vi "Dashboard Main0.vi"() -> ()   [LabVIEW 2015]
uses:
  Vision FRC Color Processing Example Folder - Copy/Vision Support Code/Camera Types.ctl
  <vilib>/Utility/miscctls.llb/LVRowAndColumnTypeDef.ctl
  <vilib>/event_ctls.llb/eventvkey.ctl
  <vilib>/Rock Robotics/Network Tables/NT Read Boolean.vi
  <vilib>/Rock Robotics/Network Tables/NT Write Boolean.vi
  <vilib>/Rock Robotics/WPI/Dashboard/WPI_DashboardLogging Global.vi
  <vilib>/Utility/config.llb/Write Key (String).vi
  <vilib>/Utility/config.llb/Write Key (I32).vi
  <vilib>/Rock Robotics/Network Tables/NT Read Numeric Array.vi
  <vilib>/Utility/config.llb/NI_LVConfig.lvlib
panel:
  out "Auton Finished 2":bool=TRUE
  in  "Camera Type":T1=enum."MS HD3000 square"
  in  "TCP":refnum<k5>
  in  "Rec Mode":enum32{"Stop", "Record", "Playback"}(radio)
  in  "Vision":u16(ring) items=["Camera Off", "USB Camera SW", "USB Camera HW", "IP Camera"]
  out "Camera IP":string
  out "Image Message":string="Timeout in Camera Communications"
  in  "Dashboard Tab":T2(tab)=enum."Custom"
  out "Shoot Now":bool=TRUE
  in  "Shoot":bool
  in  "Defense Type":T3(ring)
  out "Auton Finished":bool
  in  "Camera Switch":bool
  out "NT Connection":bool
  in  "Camera Settings":T4={"Frame Rate"=30, "Compression"=30, "Size"=1} {"Frame Rate" scale=1.0..30.0; "Size" items=["640x480", "320x240", "160x120"]}
  out "Mode":T5(ring)=enum."Auto Disabled"
  in  "DB Camera Config":bool
  out "fps":dbl format="%#.1g"
  out "Mbps":dbl format="%#.1g"
  out "Mbps LED":bool
  out "RPM":dbl(slide) scale=0.0..20000.0
  out "Arm Encoder":dbl(slide) scale=-1.0..1.0
  out "Camera Aimed":bool
  in  "Defense Location":enum16{"0", "1", "2", "3", "4", "5"}(ring)
  out "Shooter Current":dbl(graph)
  in  "DB/String 0":string
  in  "DB/Slider 1":dbl(slide) scale=0.0..5.0
  out "DB/LED 1":bool
  out "DB/LED 0":bool
  in  "DB/Button 3":bool
  in  "DB/Button 2":bool
  in  "DB/Button 1":bool caption="LED Light"
  in  "DB/Button 0":bool
  out "JS1 Z":dbl(slide) scale=-1.0..1.0 scale format="%#_2e"
  out "JS1 Graph":cluster{"X":dbl, "Y":dbl}[](graph)
  out "JS1 Buttons":T6
  out "JS2 Z":dbl(slide) scale=-1.0..1.0 scale format="%#_2e"
  out "JS2 Graph":cluster{"X":dbl, "Y":dbl}[](graph)
  out "JS2 Buttons":T6
  out "Detected Targets":T7(array[cluster]) {"Normalized Rect"."Numeric 5" format="%#_2g"; "Normalized Rect"."Numeric 3" format="%#_2g"; "Normalized Rect"."Numeric 2" format="%#_2g"; "Normalized Rect"."Numeric" format="%#_2g"}
  in  "LED Color":T8={"Hue"={51.43401092766074, 170.53085495574481}, "Sat"={34.78571428571429, 255.0}, "Val"={91.07142857142858, 255.0}} {"Hue" scale=0.0..255.0 scale format="%#_3g"}
  in  "Std Devs for Calibration":cluster{"H":dbl, "S":dbl, "V":dbl}={"H"=4.0, "S"=6.0, "V"=6.0}
  in  "Min Score Threshold":i32=20
  out "Target Distance":dbl
  out "Target X":dbl
  out "Target Y":dbl
  in  "Test Slider":dbl(slide) scale=0.0..100.0 scale format="%#_3g"
  in  "On/Off":bool caption="Solenoid"
  in  "Test Name":u16(ring) items=["Select the test to run..."]
  in  "Test Tree":string(tree)
  in  "Motor":cluster{"Value":dbl, "Enable":bool} {"Value" scale=-1.0..1.0 scale format="%#_3g"}
  out "Progress":T9 {"Test Progress" scale=0.0..100.0}
  in  "Rev/Fwd":cluster{"Forward":bool, "Reverse":bool}
  in  "Test Ring":u16(ring) items=["Monochrome", "Color"]
  out "Cmd Status":string
  in  "Execute Command":bool
  in  "Command Params":string[][](table)
  in  "Command Selection":i32(listbox)
  in  "CheckList":i32(listbox)
  out "Tree":string(tree)
  out "Camera Image":T10(plugin-control)
  out "Background":bool
  # "Right"
  # "Left"
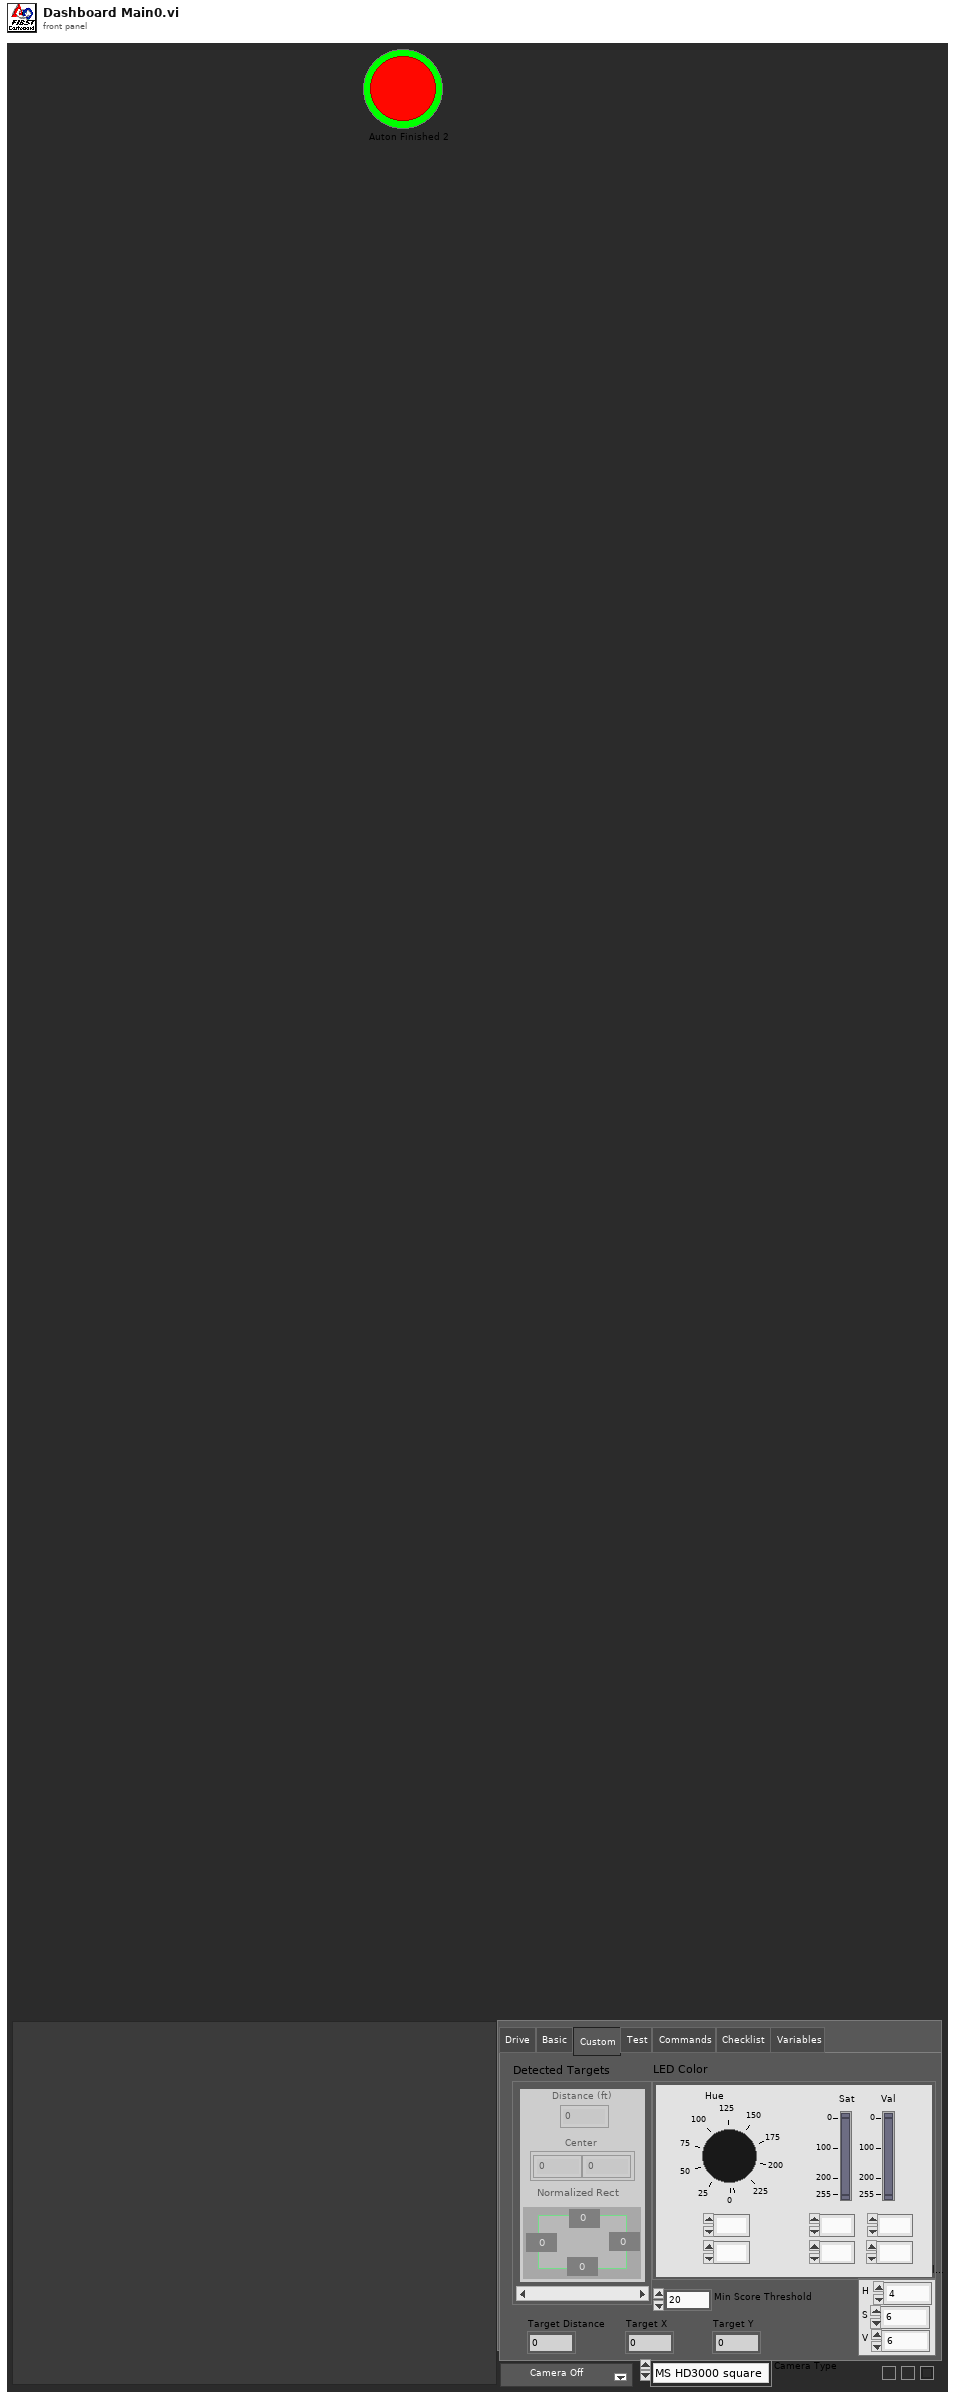
[diagram p1: front panel]
types:
  T1 = typedef "Camera Types.ctl" = enum16{"206", "1011", "1013", "MS HD3000 square", "MS HD3000 640x480"}
  T2 = enum32{"Drive", "Basic", "Custom", "Test", "Commands", "Checklist", "Variables"}
  T3 = enum16{"None", "Rampart", "Moat", "Rock Wall", "Rough Terrain", "Low Bar", "Chili Fries"}
  T4 = cluster{"Frame Rate":i32, "Compression":i32, "Size":u16}
  T5 = enum8{"Tele-Op Disabled", "Tele-Op Enabled", "Auto Disabled", "Auto Enabled", "Test Disabled", "Test Enabled", "Disconnected", "No Code", "E-Stop"}
  T6 = cluster{bool, bool, bool, bool, bool, bool, bool, bool, bool, bool, bool, bool}
  T7 = cluster{"Distance (ft)":dbl, "Center":cluster{dbl, dbl}, "Normalized Rect":cluster{"Numeric":dbl, "Numeric 2":dbl, "Numeric 3":dbl, "Numeric 5":dbl}}[]
  T8 = cluster{"Hue":cluster{dbl, dbl}, "Sat":cluster{dbl, dbl}, "Val":cluster{dbl, dbl}}
  T9 = cluster{"Test Progress":u8, "Test Progress Text":string}
  T10 = typedef "IMAQ Image.ctl" = refnum<image>
  T11 = cluster{"IDs":cluster{"RPC field ID":u16, "Unique ID":u16}, "String":string}
  T12 = enum32{"Drive", "Basic", "Custom", "Test", "Checklist", "Variables"}
  T13 = typedef "Image Type" = u32
  T14 = cluster{"Camera Image":refnum<vi>, "Dashboard Tab":refnum<vi>, "Background":refnum<vi>, "Vision":refnum<vi>, "Rec Mode":refnum<vi>, "Test Slider":refnum<vi>, "On/Off ":refnum<vi>, "Test Ring":refnum<vi>, "Rev/Fwd":refnum<vi>, "Test Name":refnum<vi>, "Motor":refnum<vi>, "Progress":refnum<vi>, "CheckList":refnum<vi>, "Tree":refnum<vi>, "Test Tree":refnum<vi>, "Command Params":refnum<vi>, "Command Selection":refnum<vi>, "Execute Command":refnum<vi>, "Cmd Status":refnum<vi>}
  T15 = typedef "NI_LVConfig.lvlib/Config Data RefNum.ctl" = refnum<k1>
  T16 = enum16{"open", "open or create", "create or replace", "create", "open (read only)"}
  T17 = cluster{"Error Strings":string, "Disable Counts":cluster{u16, u16}, "Rail Faults":cluster{u16, u16, u16}, "Robot IP":string, "DB Mode":u8, "Event Info":cluster{"Name":string, "Type":u8, "Number":u16, "Replay":u8}, "Camera Addr":string}
  T18 = cluster{"Storage":cluster{"Disk Free":u64, "RAM Block":u32, "RAM free":u32}, "CPU Utilization":cluster{"CPU % ISR":sgl, "CPU % Time Crit":sgl, "CPU % Timed Str":sgl, "CPU % High":sgl, "CPU % Above":sgl, "CPU % Normal":sgl, "CPU % Low":sgl}, "CAN":cluster{"% Bus Utilization":sgl, "Bus Off Cnt":u32, "TX_FIFO Full Cnt":u32, "Receive Error Cnt":u8, "Transmit Error Cnt":u8}, "HID":cluster{"HID Outputs":u32, "Rumble Low":u16, "Rumble High":u16}[]}
  T19 = cluster{"Status bits":cluster{"Test Mode":bool, "Autonomous":bool, "Enabled":bool, "Code Start":bool, "Brownout":bool, "Reserved 2":bool, "Reserved 3":bool, "E-Stop":bool}, "Code Trace":cluster{"Disabled":bool, "TeleOp":bool, "Auto":bool, "Test":bool}, "Controller Type":enum16{"unknown", "cRIO", "roboRio"}, "Code?":enum16{"unknown", "noCode", "code"}, "Battery V":dbl}
  T20 = cluster{"Control Bits":cluster{"TestMode":bool, "Autonomous":bool, "Enabled":bool, "FMS Present":bool, bool, bool, bool, "E-Stop":bool}, "Team Station ":u8, "Countdown":sgl, "Joystick Values":cluster{"Axes":dbl[], "Buttons":bool[], "POVs":i16[]}[]}
  T21 = cluster{"Axes":dbl[], "Buttons":bool[], "POVs":i16[]}[]
  T22 = cluster{"Test Mode":bool, "Autonomous":bool, "Enabled":bool, "Code Start":bool, "Brownout":bool, "Reserved 2":bool, "Reserved 3":bool, "E-Stop":bool}
  T23 = cluster{"Axes":dbl[], "Buttons":bool[], "POVs":i16[]}
  T24 = cluster{"Buttons[0]":bool, "Buttons[1]":bool, "Buttons[2]":bool, "Buttons[3]":bool, "Buttons[4]":bool, "Buttons[5]":bool, "Buttons[6]":bool, "Buttons[7]":bool, "Buttons[8]":bool, "Buttons[9]":bool, "Buttons[10]":bool, "Buttons[11]":bool}
  T25 = cluster{"Detected Targets[0]":cluster{"Distance (ft)":dbl, "Center":cluster{dbl, dbl}, "Normalized Rect":cluster{"Numeric":dbl, "Numeric 2":dbl, "Numeric 3":dbl, "Numeric 5":dbl}}, "Detected Targets[1]":cluster{"Distance (ft)":dbl, "Center":cluster{dbl, dbl}, "Normalized Rect":cluster{"Numeric":dbl, "Numeric 2":dbl, "Numeric 3":dbl, "Numeric 5":dbl}}, "Detected Targets[2]":cluster{"Distance (ft)":dbl, "Center":cluster{dbl, dbl}, "Normalized Rect":cluster{"Numeric":dbl, "Numeric 2":dbl, "Numeric 3":dbl, "Numeric 5":dbl}}, "Detected Targets[3]":cluster{"Distance (ft)":dbl, "Center":cluster{dbl, dbl}, "Normalized Rect":cluster{"Numeric":dbl, "Numeric 2":dbl, "Numeric 3":dbl, "Numeric 5":dbl}}, "Detected Targets[4]":cluster{"Distance (ft)":dbl, "Center":cluster{dbl, dbl}, "Normalized Rect":cluster{"Numeric":dbl, "Numeric 2":dbl, "Numeric 3":dbl, "Numeric 5":dbl}}, "Detected Targets[5]":cluster{"Distance (ft)":dbl, "Center":cluster{dbl, dbl}, "Normalized Rect":cluster{"Numeric":dbl, "Numeric 2":dbl, "Numeric 3":dbl, "Numeric 5":dbl}}, "Detected Targets[6]":cluster{"Distance (ft)":dbl, "Center":cluster{dbl, dbl}, "Normalized Rect":cluster{"Numeric":dbl, "Numeric 2":dbl, "Numeric 3":dbl, "Numeric 5":dbl}}, "Detected Targets[7]":cluster{"Distance (ft)":dbl, "Center":cluster{dbl, dbl}, "Normalized Rect":cluster{"Numeric":dbl, "Numeric 2":dbl, "Numeric 3":dbl, "Numeric 5":dbl}}, "Detected Targets[8]":cluster{"Distance (ft)":dbl, "Center":cluster{dbl, dbl}, "Normalized Rect":cluster{"Numeric":dbl, "Numeric 2":dbl, "Numeric 3":dbl, "Numeric 5":dbl}}}
  T26 = cluster{"Distance (ft)":dbl, "Center":cluster{dbl, dbl}, "Normalized Rect":cluster{"Numeric":dbl, "Numeric 2":dbl, "Numeric 3":dbl, "Numeric 5":dbl}}
  T27 = cluster{"Numeric":dbl, "Numeric 2":dbl, "Numeric 3":dbl, "Numeric 5":dbl}
  T28 = cluster{"Operation":enum16{"Update", "Clear"}, "Color Box":u32}[]
  T29 = typedef "eventvkey.ctl" = enum16{"ASCII", "Enter", "Return", "Shift", "Ctrl", "Alt", "Cmd", "Opt", "Caps", "NumLock", "Clear", "Break", "Up", "Down", "Left", "Right", "Insert", "Delete", "Home", "End", "PageUp", "PageDown", "Escape", "Help", "Pause", "ScrollLock", "F1", "F2", "F3", "F4", "F5", "F6", "F7", "F8", "F9", "F10", "F11", "F12", "F13", "F14", "F15", "F16", "F17", "F18", "F19", "F20", "F21", "F22", "F23", "F24", "Play", "VolumeUp", "VolumeDown", "Mute", "Two Byte Char"}
  T30 = cluster{"Image Size":bool, "Image Type":bool, "Pixel Value":bool, "ROI Information":bool, "Zoom Factor":bool}
  T31 = enum8{"Enabled", "Disabled", "Disabled and Grayed Out"}
  T32 = cluster{"Operation":enum16{"Update", "Clear"}, "Color Box":u32}
  T33 = typedef "LVRowAndColumnTypeDef.ctl" = cluster{"Row":i32, "Column":i32}
  T34 = cluster{"Shift":bool, "Ctrl":bool, "Alt":bool, "Cmd":bool, "Opt":bool}
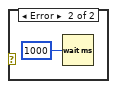
[diagram p2: hidden frame]
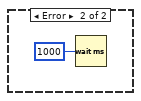
[diagram p3: hidden frame]
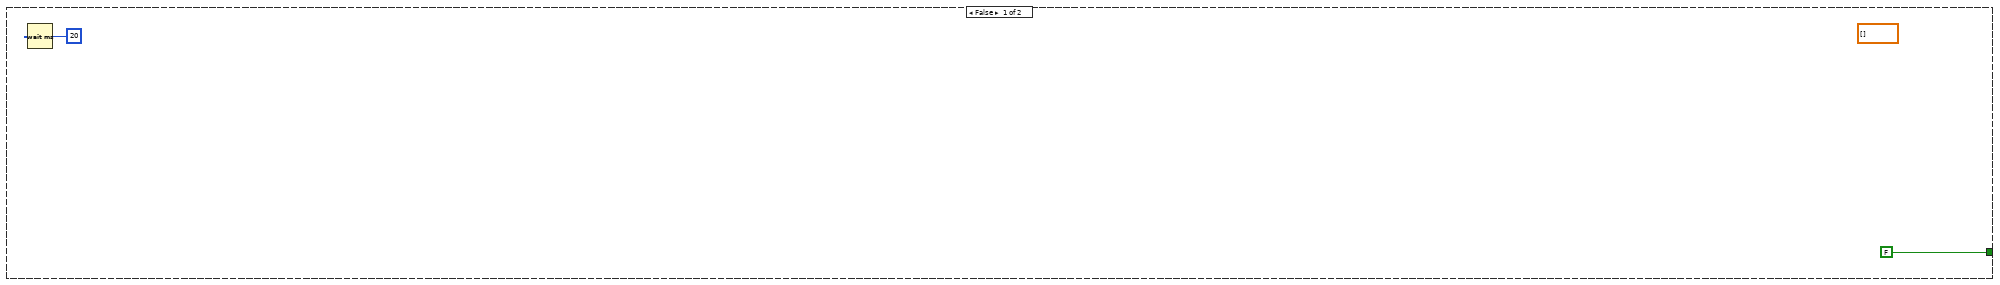
[diagram p4: hidden frame]
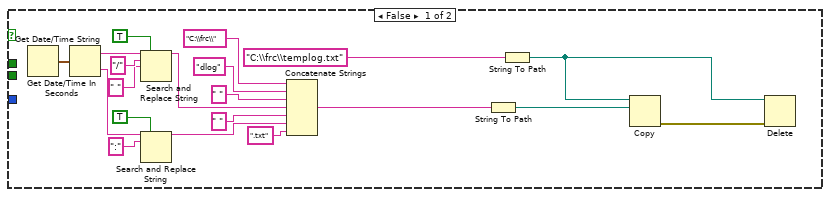
[diagram p5: hidden frame]
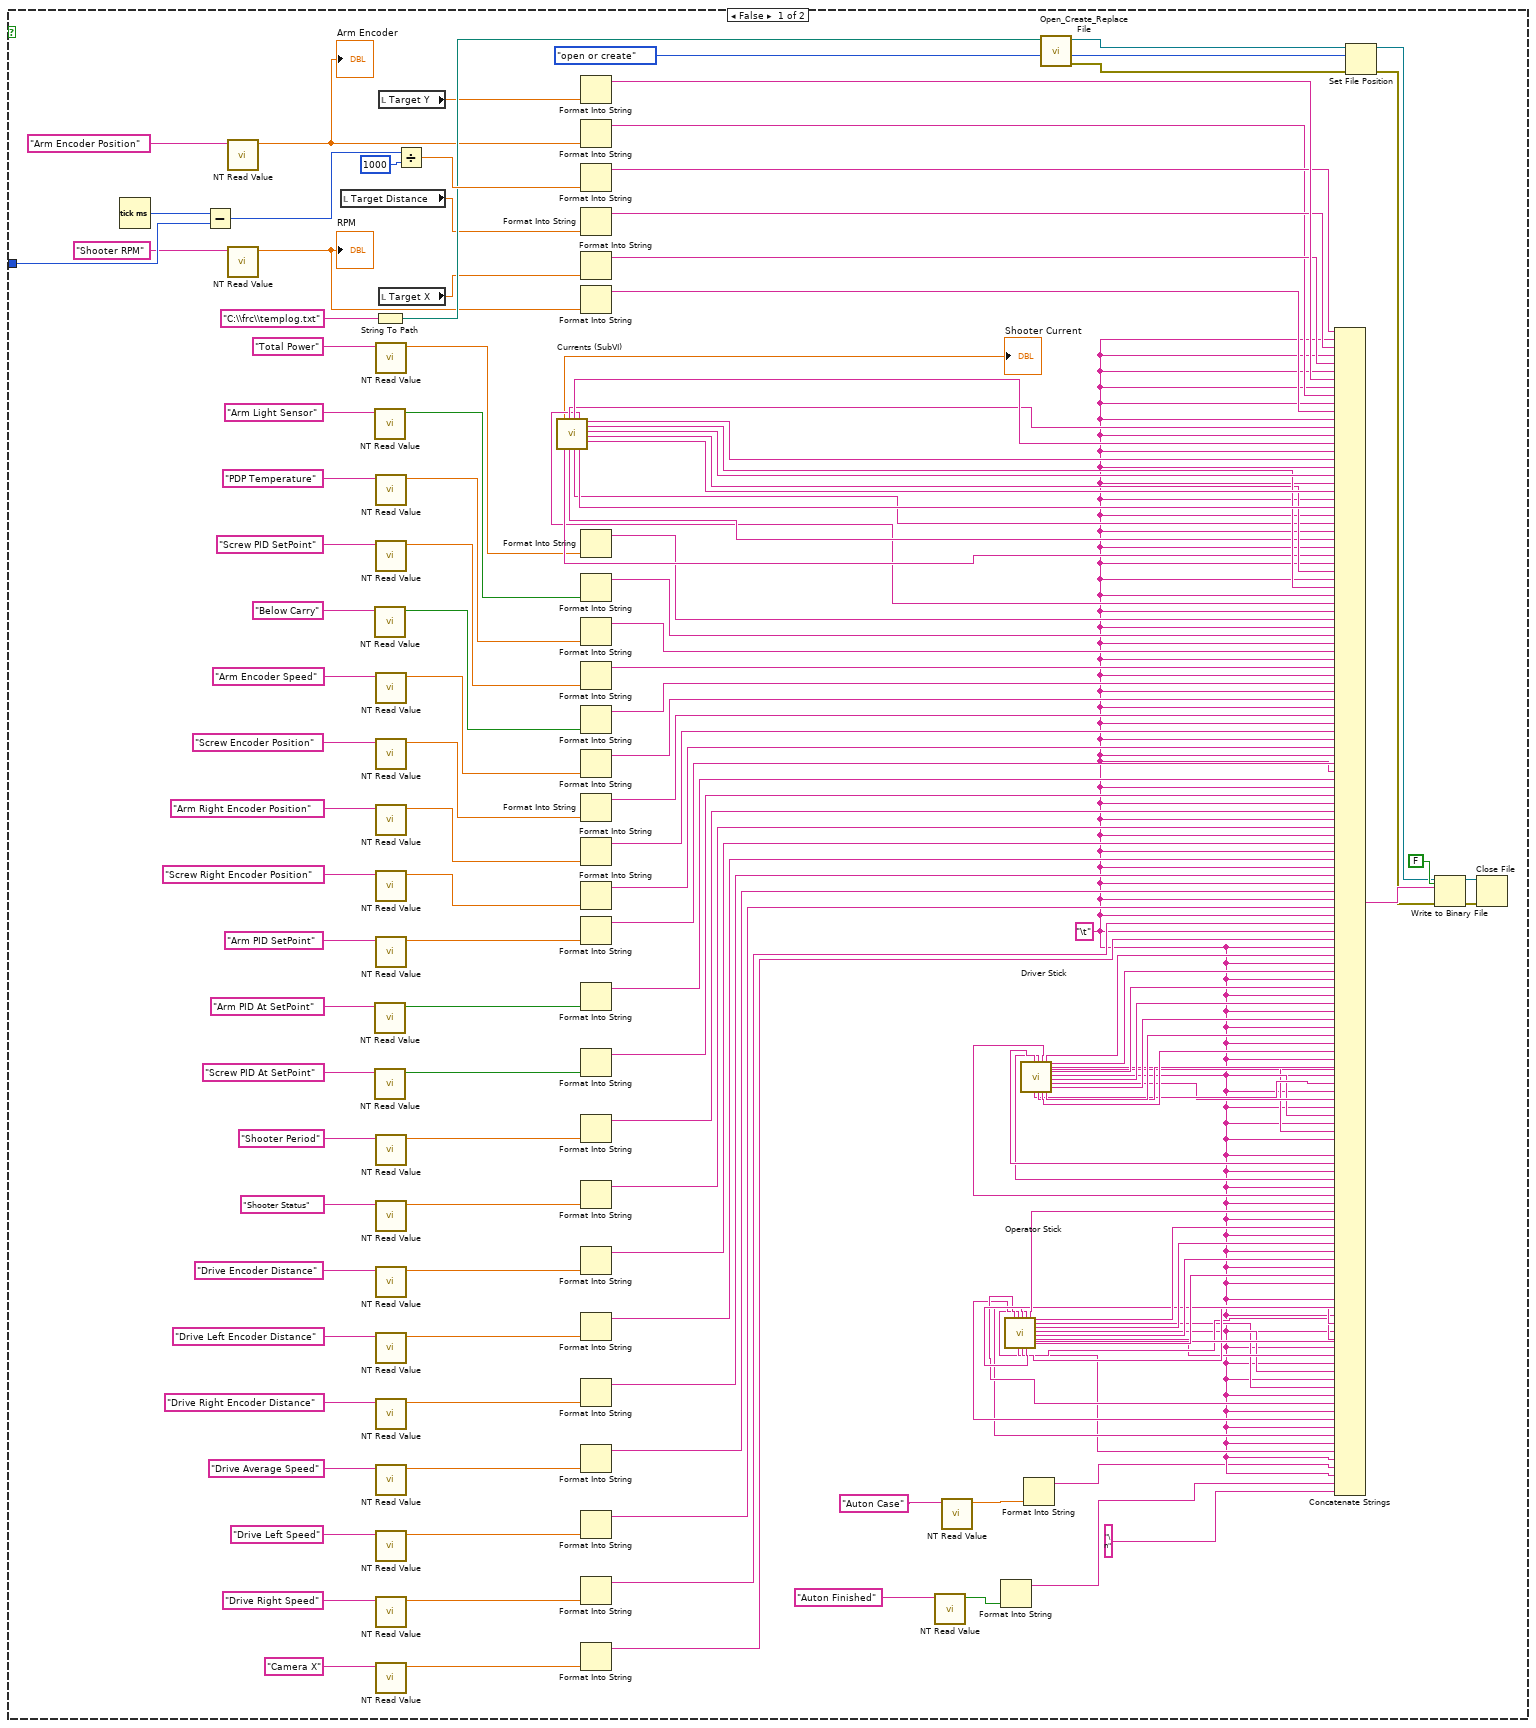
[diagram p6: hidden frame]
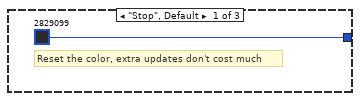
[diagram p7: hidden frame]
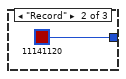
[diagram p8: hidden frame]
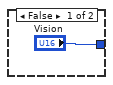
[diagram p10: hidden frame]
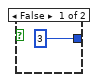
[diagram p11: hidden frame]
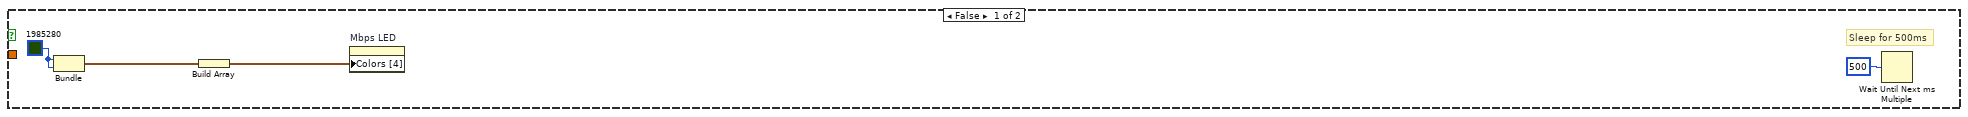
[diagram p12: hidden frame]
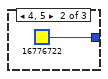
[diagram p13: hidden frame]
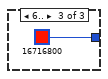
[diagram p14: hidden frame]
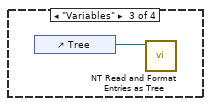
[diagram p16: hidden frame]
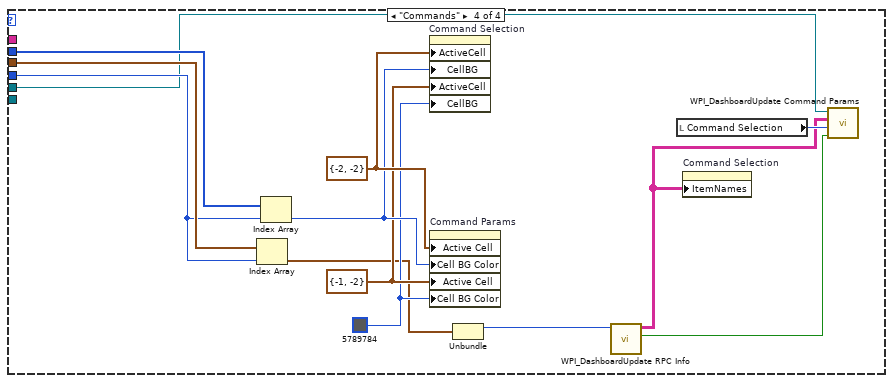
[diagram p17: hidden frame]
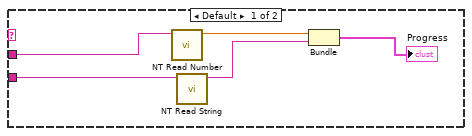
[diagram p18: hidden frame]
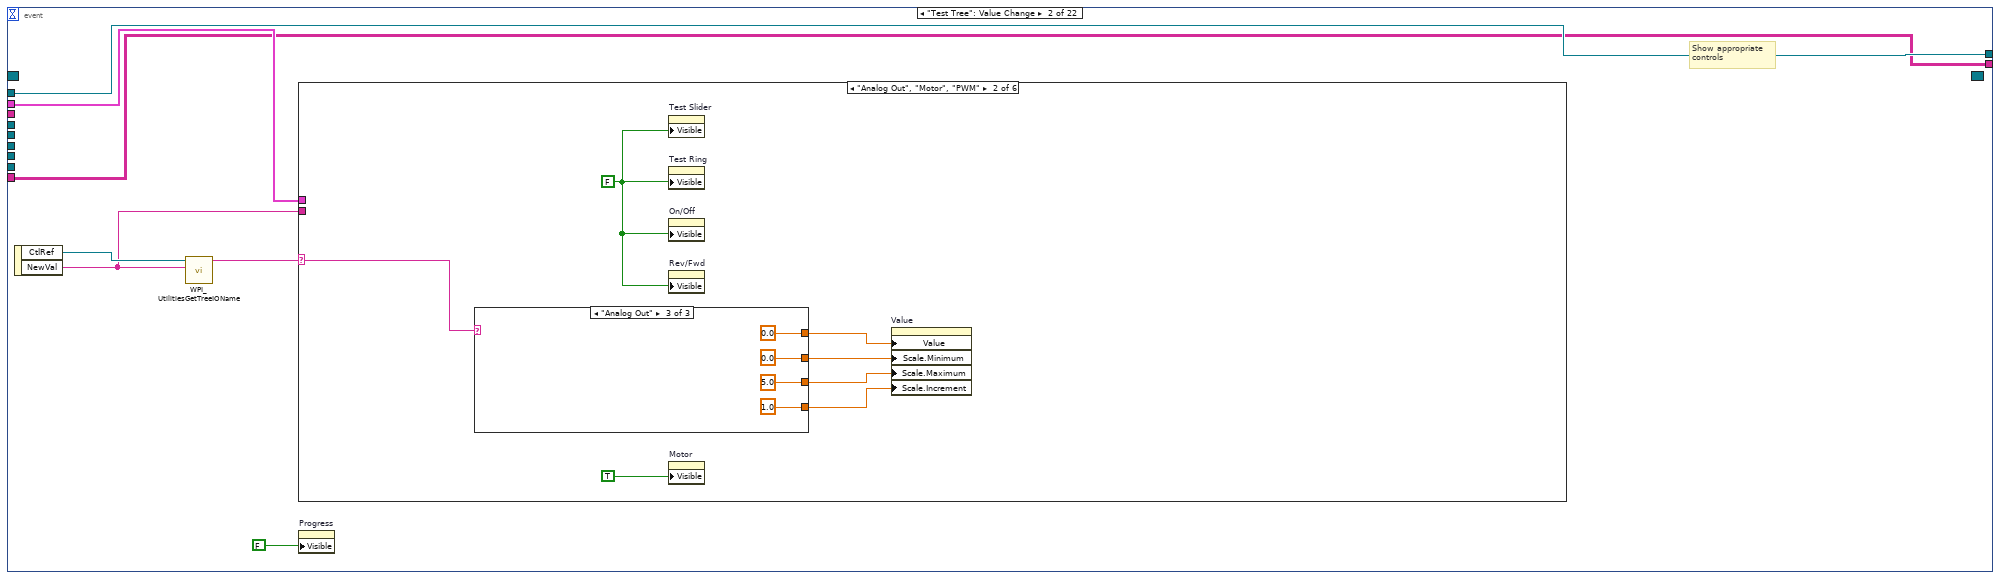
[diagram p19: hidden frame]
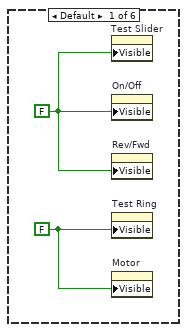
[diagram p20: hidden frame]
diagram:
  w10 = T11 {"IDs"={"RPC field ID"=0, "Unique ID"=0}, "String"=""}  # RPC Response
  w34 = 491  # min tab size
  w33 = 1.333  # min tab size
  w42 = enum32{"Stop", "Record", "Playback"}."Stop" ("Rec Mode")
  w16 = FALSE ("Visible")
  (unwired) "This VI has seven parallel loops for different tasks and a bit of initialization code that runs just once.\n\nTypical dashboard extensions only need to edit the panel. Adding new indicators or controls simply involves placing them on the panel in the Operations tab and naming them the same as the SmartDashboard variable on the robot\n\nIf the display needs to process the data before display, loop one is an example of doing that for the joysticks and motors.\n\nIf you want customize the video display or perform processing on it, loop two is where that takes place.\n\nOther loops should not need to be modified. They are pretty standard, and document the task they perform."  # Documentation
  w62 = T13 4 items=["Grayscale (U8)", "Grayscale (I16)", "Grayscale (SGL)", "Complex (CSG)", "RGB (U32)", "HSL (U32)", "RGB (U64)"] ("Image Type")
  # "Loop 7. Wait for DS connections"
  # "Basic debug and auto controls: Their data names are fixed, but\nthe displayed name, called a caption, can be changed directly or in\nrobot code such as shown in Begin."
  # "Controls for Test Mode, Camera Settings, etc."
  # "Additional UI Initialization"
  # "Loop 6. Animation for background of window during playback and record"
  # "Fires each time robot IP\nchanges, simulator does this"
  # "Fires each time window\ndocking changes."
  # "Collects all controls and indicators\nin the Basic and Custom tab.\nIf you need to bind additional controls,\nadd their references. You can extend the\nenum constant or use an integer."
  # "The remaining code below this line typically doesn't need to be modified."
  # "Loop 4. Process UI events related to test mode, checklist, and camera settings"
  # "Terminals of controls and indicators that are bound to the smart dashboard by name.\nYou can place the terminals anywhere you like and even read data from them.\nYou bind controls by adding the control reference to the array on the left. The subVI will\ndo this for the contents of a tab, and you can do it for individual items too, as shown with\nthe LED. To create get the reference, right-click and Create>>Reference."
  # "Loop 3. Wait until the robot response provides\n the Robot IP address.\nOnce known, bind controls and\nvariables with the same names."
  # "Loop 5. Adjusts placement onscreen, hides the titlebar, etc."
  # "Loop 1. Receive various data streams from Driver Station, update joystick, motors, and more complex displays that don't easily bind to variables."
  # "Loop 2. Receive camera images from Robot, update Mbps, fps, and do any processing or display"
  n1 = control-ref of="Dashboard Tab"() -> (w40:refnum<vi>)
  n2 = control-ref of="Rec Mode"() -> (w22:refnum<vi>)
  n3 = control-ref of="Command Selection"() -> (w9:refnum<vi>)
  n4 = control-ref of="Command Params"() -> (w12:refnum<vi>)
  n5 = control-ref of="Execute Command"() -> (w11:refnum<vi>)
  n6 = control-ref of="Camera Image"() -> (w37:refnum<vi>)
  n7 = call "IMAQ Create"("Image Name"="Dashboard Image", "Image Type"=w62) -> ("New Image"=w60:T10, "error out"=w59:errorcluster)  [unwired: 2 in, 1 out]
  n8 = control-ref of="Dashboard Tab"() -> (w36:refnum<vi>)
  n9 = control-ref of="Tree"() -> (w26:refnum<vi>)
  n10 = control-ref of="Test Tree"() -> (w25:refnum<vi>)
  n11 = control-ref of="Background"() -> (w31:refnum<vi>)
  n12 = control-ref of="Cmd Status"() -> (w5:refnum<vi>)
  n13 = control-ref of="On/Off"() -> (w20:refnum<vi>)
  n14 = control-ref of="Test Name"() -> (w24:refnum<vi>)
  n15 = control-ref of="Command Params"() -> (w4:refnum<vi>)
  n16 = control-ref of="Test Slider"() -> (w21:refnum<vi>)
  n17 = control-ref of="Rev/Fwd"() -> (w18:refnum<vi>)
  n18 = control-ref of="Motor"() -> (w23:refnum<vi>)
  n19 = control-ref of="Progress"() -> (w17:refnum<vi>)
  n20 = control-ref of="CheckList"() -> (w27:refnum<vi>)
  n21 = control-ref of="Test Ring"() -> (w19:refnum<vi>)
  n22 = Obtain Notifier(name (unnamed)="Window Mode", notification data type=TRUE) -> (notifier out=w3:refnum<notifier>)  [unwired: 2 in, 2 out]
  n23 = call <vilib>:"Get Tab Control Refs.vi"("Page Index"=T12."Basic" ("Dashboard Tab"), "TabControl in"=w40) -> ("ControlsOnPage"=w15:refnum<vi>[])  [unwired: 9 in]
  n24 = call <vilib>:"Get Tab Control Refs.vi"("Page Index"=T12."Custom" ("Dashboard Tab"), "TabControl in"=w40) -> ("ControlsOnPage"=w39:refnum<vi>[])  [unwired: 9 in]
  n25 = control-ref of="Vision"() -> (w35:refnum<vi>)
  n26 = Bundle("min tab size"=w34, "min tab size"=w33) -> (w32:cluster{"min tab size":i32, "min tab size":dbl})  [unwired: 1 in]
  n27 = Obtain Notifier(name (unnamed)="Robot IP Update", notification data type="IP Addr" ("name (unnamed)")) -> (notifier out=w2:refnum<notifier>)  [unwired: 2 in, 2 out]
  n28 = property class="VI" props=["Front Panel.Closeable"]() -> (reference out=w41:refnum<vi>)  [unwired: 2 in, 2 out]
  n29 = vi-ref "Playback Controls.vi"() -> (w47:refnum<vi>)
  n30 = Build Array (concatenate)(w15, w39) -> (w38:refnum<vi>[])
  n31 = Bundle("Camera Image"=w37, "Dashboard Tab"=w36, "Background"=w31, "Vision"=w35, "Rec Mode"=w22, "Test Slider"=w21, "On/Off"=w20, "Test Ring"=w19, "Rev/Fwd"=w18, "Test Name"=w24, "Motor"=w23, "Progress"=w17, "CheckList"=w27, "Tree"=w26, "Test Tree"=w25, "Command Params"=w12, "Command Selection"=w9, "Execute Command"=w11, "Cmd Status"=w5) -> (w28:T14)  [unwired: 1 in]
  n32 = Create User Event(user event datatype=w10) -> (user event=w6:refnum<user-event>)  [unwired: 1 in, 1 out]
  n33 = call "Adjust Dashboard Window.vi"("Sizing Refnums"=w28, "Size Constraints"=w32, "VI"=w41, "WIn Mode"=w3) -> ()  [unwired: 8 in]
  n34 = while {
    tunnel: w38 -> [w75]
    tunnel: w2 -> [w73]
    tunnel: [w71] -> _
    tunnel: u32 1000 ("milliseconds to wait") -> [w70]
    tunnel: w6 -> [w63]
    i -> [w71]
    stop <- FALSE stop-if-true
    n35 = local read "Rec Mode"() -> (w66:enum32{"Stop", "Record", "Playback"})
    n36 = Wait on Notification(notifier=w73, timeout in ms (-1)=w70) -> (notification=w72:string, timed out?=w68:bool)  [unwired: 2 in, 2 out]
    n37 = Equal?(x=w66, y=u16 2 ("Rec Mode")) -> (x = y?=w67:bool)
    n38 = Compound Arithmetic op=OR(invert w68, w67) -> (w69:bool)
    n39 = case shown="True" w69 {
      tunnel: w75 -> [_ w79]
      tunnel: w72 -> [_ w78]
      tunnel: "Dashboard" -> [_ w77]
      tunnel: w63 -> [_ w76]
      frame False {
      }
      frame True {
        n40 = call <vilib>:"Bind Controls to SmartDashboard.vi"("RPC ref"=w76, "Client Name"=w77, "Bound Control Refs"=w79, "Server IP Address"=w78) -> ()  [unwired: 8 in]
      }
    }
  }
  n41 = register-events(refnum<vi> refnum, w6) -> (reference out=w46:refnum<event-registration>, error out=w45:errorcluster)  [unwired: 2 in]
  n42 = property class="VI"() -> ("Panel"=w49:refnum<vi>)  [unwired: 2 in, 2 out]
  n43 = call "Initialize Camera and CheckList.vi"("ListBox in"=w27) -> ("Cluster"=w53:cluster{"value":i32, "value":i32, "index":i32}, "Array"=w54:cluster{string[]}[], "File Refnum"=w52:T15)  [unwired: 8 in]
  n44 = property class="Pnl"(reference=w49) -> ("Panes[]"=w50:refnum<vi>[])  [unwired: 1 in, 2 out]
  n45 = property on="Camera Settings" class="Clust (strict)"("Val(Sgnl)"=w53) -> ()  [unwired: 2 in, 2 out]
  n46 = Tick Count (ms)() -> (millisecond timer value=w1:u32)
  n47 = control-ref of="Test Tree"() -> (w51:refnum<vi>)
  n48 = Index Array(array=w50) -> (element=w48:refnum<vi>)  [unwired: 1 in]
  n49 = while {
    tunnel: w48 -> [w81]
    i -> [w84]
    stop <- FALSE stop-if-true
    n50 = Wait (ms)(milliseconds to wait=u32 100) -> ()  [unwired: 1 out]
    n51 = case shown="\"Playback\"" "Rec Mode" {
      tunnel: w84 -> [_ _ w99]
      tunnel: [u32 2829099 ("Base Color") u32 11141120 ("Target Color") w88] -> w80
      frame "Stop", Default {
        # "Reset the color, extra updates don't cost much"
      }
      frame "Record" {
      }
      frame "Playback" {
        # "Playback"
        n52 = Quotient & Remainder(x=w99, y=u32 50 ("milliseconds to wait")) -> (x-y*floor(x/y)=w95:u32)  [unwired: 1 out]
        n53 = Divide(x=w95, y=u32 50 ("milliseconds to wait")) -> (x/y=w92:dbl)
        n54 = Multiply(x=6.283185307179586, y=w92) -> (x*y=w97:dbl)
        n55 = Sine(x=w97) -> (sin(x)=w96:dbl)
        n56 = Absolute Value(x=w96) -> (abs(x)=w89:dbl)
        n57 = call "Interpolate RGB Color.vi"("Proportion"=w89, "Target Color"=u32 30976, "Base Color"=u32 2829099) -> ("Result Color"=w88:u32)  [unwired: 8 in]
      }
    }
    n58 = property class="Pane"(reference=w81, "PaneColor"=w80) -> ()  [unwired: 1 in, 2 out]
  }
  n59 = while {
    tunnel: [w114] -> _
    tunnel: w2 -> [w108]
    tunnel: w15 -> [w107]
    tunnel: w3 -> [w103]
    tunnel: w1 -> [w102]
    shift-right: [w101] -> _
    shift-left: _ -> [w100]
    i -> [w114]
    stop <- FALSE stop-if-true
    n60 = call <vilib>:"WPI_DashboardUpdateNames.vi"("Controls on Tab"=w107) -> ()  [unwired: 11 in]
    n61 = local read "Vision"() -> (w105:u16)
    n62 = call <vilib>:"WPI_DashboardRetrieveStatusInfo.vi"("Vision"=w105, "Binding Refnum"=w108, "Window Mode Notifier"=w103, "TCP Cnx"="TCP") -> ("Power and Errors"=w109:T17, "Robot Metrics"=w112:T18, "Status Info"=w113:T19, "Control Info"=w110:T20, "Robot Mode"=w106:T5, "Process?"=w111:bool)  [unwired: 2 in]
    "Mode" <- w106
    n63 = case shown="True" w111 {
      tunnel: w113 -> [_ w143]
      tunnel: w112 -> [_ w142]
      tunnel: w110 -> [_ w141]
      tunnel: w109 -> [_ w140]
      tunnel: w106 -> [_ _]
      tunnel: w102 -> [_ w124]
      tunnel: [FALSE ("Enabled") w122] -> w101
      tunnel: w100 -> [_ w123]
      frame False {
        (unwired) dbl[] []
        n64 = Wait (ms)(milliseconds to wait=u32 20) -> ()  [unwired: 1 out]
      }
      frame True {
        # "swap motors to match\ncharts and include battery"
        n65 = Unbundle By Name(w141) -> ("Joystick Values"=w137:T21)  [unwired: 5 out]
        n66 = Unbundle By Name(w142) -> ()  [unwired: 5 out]
        n67 = Unbundle By Name(w140) -> ("Camera Addr"=→"Camera IP":string)  [unwired: 4 out]
        n68 = Unbundle By Name(w143) -> ("Status bits"=w125:T22)  [unwired: 1 out]
        n69 = Unbundle By Name(w125) -> ("Enabled"=w122:bool)  [unwired: 7 out]
        n70 = Index Array(array=w137) -> (element #1=w136:T23, element #2=w131:T23)  [unwired: 2 in]
        n71 = case shown="True" w122 {
          tunnel: w124 -> [_ w167]
          tunnel: w123 -> [_ w165]
          tunnel: w122 -> [_ w164]
          frame False {
            n72 = Get Date/Time In Seconds() -> (seconds since 1Jan1904=w156:timestamp)
            n73 = Get Date/Time String(seconds (now)=w156) -> (date string=w154:string, time string=w155:string)  [unwired: 2 in]
            n74 = Search and Replace String(replace all?=TRUE ("replace all? (F)"), input string=w154, search string="/", replace string=" " ("replace string (\"\")")) -> (result string=w147:string)  [unwired: 4 in, 3 out]
            n75 = Search and Replace String(replace all?=TRUE ("replace all? (F)"), input string=w155, search string=":") -> (result string=w145:string)  [unwired: 5 in, 3 out]
            n76 = Concatenate Strings("C:\\frc\\" ("string"), "dlog" ("string"), " " ("string"), w147, " " ("string"), w145, ".txt" ("string")) -> (w159:string)
            n77 = String To Path(string=w159) -> (path=w160:path)
            n78 = String To Path(string="C:\\frc\\templog.txt") -> (path=w161:path)
            n79 = Copy(10:w160, 11:w161) -> (0:w162:errorcluster)  [unwired: 3 in, 2 out]
            n80 = Delete(path (use dialog)=w161, error in=w162) -> ()  [unwired: 3 in, 3 out]
          }
          frame True {
            n81 = Not Equal?(x=w164, y=w165) -> (x != y?=w166:bool)
            n82 = case shown="True" w166 {
              tunnel: w167 -> [w281 _]
              frame False {
                w170 = "\t" ("string")
                n83 = Tick Count (ms)() -> (millisecond timer value=w283:u32)
                n84 = Subtract(x=w283, y=w281) -> (x-y=w282:u32)
                n85 = call-poly <vilib>:"NT Read Value.vi"("Name"="Arm Encoder Position") -> ("Numeric"=w276:dbl)  [unwired: 9 in, 1 out]
                "Arm Encoder" <- w276
                n86 = call-poly <vilib>:"NT Read Value.vi"("Name"="Shooter RPM") -> ("Numeric"=w273:dbl)  [unwired: 9 in, 1 out]
                "RPM" <- w273
                n87 = local read "Target Distance"() -> (w280:dbl)
                n88 = String To Path(string="C:\\frc\\templog.txt") -> (path=w293:path)
                n89 = call-poly <vilib>:"NT Read Value.vi"("Name"="Arm Light Sensor") -> ("Boolean"=w197:bool)  [unwired: 9 in, 1 out]
                n90 = call-poly <vilib>:"NT Read Value.vi"("Name"="Below Carry") -> ("Boolean"=w254:bool)  [unwired: 9 in, 1 out]
                n91 = call-poly <vilib>:"NT Read Value.vi"("Name"="Arm PID At SetPoint") -> ("Boolean"=w244:bool)  [unwired: 9 in, 1 out]
                n92 = call-poly <vilib>:"NT Read Value.vi"("Name"="Screw PID At SetPoint") -> ("Boolean"=w240:bool)  [unwired: 9 in, 1 out]
                n93 = call-poly <vilib>:"NT Read Value.vi"("Name"="Total Power") -> ("Numeric"=w269:dbl)  [unwired: 9 in, 1 out]
                n94 = call-poly <vilib>:"NT Read Value.vi"("Name"="PDP Temperature") -> ("Numeric"=w267:dbl)  [unwired: 9 in, 1 out]
                n95 = call-poly <vilib>:"NT Read Value.vi"("Name"="Screw PID SetPoint") -> ("Numeric"=w271:dbl)  [unwired: 9 in, 1 out]
                n96 = call-poly <vilib>:"NT Read Value.vi"("Name"="Arm Encoder Speed") -> ("Numeric"=w256:dbl)  [unwired: 9 in, 1 out]
                n97 = call-poly <vilib>:"NT Read Value.vi"("Name"="Screw Encoder Position") -> ("Numeric"=w260:dbl)  [unwired: 9 in, 1 out]
                n98 = call-poly <vilib>:"NT Read Value.vi"("Name"="Arm Right Encoder Position") -> ("Numeric"=w258:dbl)  [unwired: 9 in, 1 out]
                n99 = call-poly <vilib>:"NT Read Value.vi"("Name"="Screw Right Encoder Position") -> ("Numeric"=w248:dbl)  [unwired: 9 in, 1 out]
                n100 = call-poly <vilib>:"NT Read Value.vi"("Name"="Arm PID SetPoint") -> ("Numeric"=w265:dbl)  [unwired: 9 in, 1 out]
                n101 = call-poly <vilib>:"NT Read Value.vi"("Name"="Shooter Period") -> ("Numeric"=w242:dbl)  [unwired: 9 in, 1 out]
                n102 = call-poly <vilib>:"NT Read Value.vi"("Name"="Shooter Status") -> ("Numeric"=w238:dbl)  [unwired: 9 in, 1 out]
                n103 = call-poly <vilib>:"NT Read Value.vi"("Name"="Drive Encoder Distance") -> ("Numeric"=w236:dbl)  [unwired: 9 in, 1 out]
                n104 = call-poly <vilib>:"NT Read Value.vi"("Name"="Drive Left Encoder Distance") -> ("Numeric"=w230:dbl)  [unwired: 9 in, 1 out]
                n105 = call-poly <vilib>:"NT Read Value.vi"("Name"="Drive Right Encoder Distance") -> ("Numeric"=w228:dbl)  [unwired: 9 in, 1 out]
                n106 = call-poly <vilib>:"NT Read Value.vi"("Name"="Drive Average Speed") -> ("Numeric"=w226:dbl)  [unwired: 9 in, 1 out]
                n107 = call-poly <vilib>:"NT Read Value.vi"("Name"="Drive Left Speed") -> ("Numeric"=w216:dbl)  [unwired: 9 in, 1 out]
                n108 = call-poly <vilib>:"NT Read Value.vi"("Name"="Drive Right Speed") -> ("Numeric"=w218:dbl)  [unwired: 9 in, 1 out]
                n109 = call-poly <vilib>:"NT Read Value.vi"("Name"="Camera X") -> ("Numeric"=w220:dbl)  [unwired: 9 in, 1 out]
                n110 = local read "Target Y"() -> (w278:dbl)
                n111 = local read "Target X"() -> (w279:dbl)
                n112 = Divide(x=w282, y=u32 1000) -> (x/y=w297:dbl)
                n113 = call "Currents (SubVI).vi"() -> ("Shooter Current"=→"Shooter Current":dbl, "String 5"=w302:string, "lf drive I"=w309:string, "String 4"=w301:string, "lr drive I"=w310:string, "String 3"=w300:string, "String"=w272:string, "String 9"=w312:string, "String 2"=w299:string, "String 7"=w304:string, "String 10"=w313:string, "String 6"=w303:string, "String 8"=w311:string)  [unwired: 7 in]
                n114 = Format Into String(w278) -> (resulting string=w308:string)  [unwired: 3 in, 1 out]
                n115 = Format Into String(w276) -> (resulting string=w275:string)  [unwired: 3 in, 1 out]
                n116 = Format Into String(w297) -> (resulting string=w306:string)  [unwired: 3 in, 1 out]
                n117 = Format Into String(w280) -> (resulting string=w298:string)  [unwired: 3 in, 1 out]
                n118 = Format Into String(w279) -> (resulting string=w307:string)  [unwired: 3 in, 1 out]
                n119 = Format Into String(w273) -> (resulting string=w274:string)  [unwired: 3 in, 1 out]
                n120 = Format Into String(w269) -> (resulting string=w263:string)  [unwired: 3 in, 1 out]
                n121 = Format Into String(w197) -> (resulting string=w195:string)  [unwired: 3 in, 1 out]
                n122 = Format Into String(w267) -> (resulting string=w262:string)  [unwired: 3 in, 1 out]
                n123 = Format Into String(w271) -> (resulting string=w261:string)  [unwired: 3 in, 1 out]
                n124 = Format Into String(w254) -> (resulting string=w252:string)  [unwired: 3 in, 1 out]
                n125 = Format Into String(w256) -> (resulting string=w251:string)  [unwired: 3 in, 1 out]
                n126 = Format Into String(w260) -> (resulting string=w250:string)  [unwired: 3 in, 1 out]
                n127 = Format Into String(w258) -> (resulting string=w249:string)  [unwired: 3 in, 1 out]
                n128 = Format Into String(w248) -> (resulting string=w246:string)  [unwired: 3 in, 1 out]
                n129 = Format Into String(w265) -> (resulting string=w245:string)  [unwired: 3 in, 1 out]
                n130 = Format Into String(w244) -> (resulting string=w234:string)  [unwired: 3 in, 1 out]
                n131 = Format Into String(w240) -> (resulting string=w233:string)  [unwired: 3 in, 1 out]
                n132 = Format Into String(w242) -> (resulting string=w232:string)  [unwired: 3 in, 1 out]
                n133 = Format Into String(w238) -> (resulting string=w231:string)  [unwired: 3 in, 1 out]
                n134 = Format Into String(w236) -> (resulting string=w224:string)  [unwired: 3 in, 1 out]
                n135 = Format Into String(w230) -> (resulting string=w223:string)  [unwired: 3 in, 1 out]
                n136 = Format Into String(w228) -> (resulting string=w222:string)  [unwired: 3 in, 1 out]
                n137 = Format Into String(w226) -> (resulting string=w221:string)  [unwired: 3 in, 1 out]
                n138 = Format Into String(w216) -> (resulting string=w214:string)  [unwired: 3 in, 1 out]
                n139 = Format Into String(w218) -> (resulting string=w213:string)  [unwired: 3 in, 1 out]
                n140 = Format Into String(w220) -> (resulting string=w212:string)  [unwired: 3 in, 1 out]
                n141 = call-poly <vilib>:"NT Read Value.vi"("Name"="Auton Finished") -> ("Boolean"=w172:bool)  [unwired: 9 in, 1 out]
                n142 = call-poly <vilib>:"NT Read Value.vi"("Name"="Auton Case") -> ("Numeric"=w174:dbl)  [unwired: 9 in, 1 out]
                n143 = Format Into String(w172) -> (resulting string=w168:string)  [unwired: 3 in, 1 out]
                n144 = call "Operator Stick.vi"() -> ("String 4"=w180:string, "String 3"=w179:string, "String 8"=w186:string, "String 2"=w178:string, "String 9"=w187:string, "String"=w177:string, "String 10"=w188:string, "String 16"=w194:string, "String 11"=w189:string, "String 15"=w193:string, "String 5"=w183:string, "String 14"=w192:string, "String 6"=w184:string, "String 13"=w191:string, "String 7"=w185:string, "String 12"=w190:string)  [unwired: 12 in]
                n145 = call "Driver Stick.vi"() -> ("String 4"=w199:string, "String 3"=w182:string, "String 8"=w203:string, "String 2"=w181:string, "String 9"=w204:string, "String"=w198:string, "String 10"=w205:string, "String 16"=w211:string, "String 11"=w206:string, "String 15"=w210:string, "String 5"=w200:string, "String 14"=w209:string, "String 6"=w201:string, "String 13"=w208:string, "String 7"=w202:string, "String 12"=w207:string)  [unwired: 12 in]
                n146 = Format Into String(w174) -> (resulting string=w169:string)  [unwired: 3 in, 1 out]
                n147 = call <vilib>:"Open_Create_Replace File.vi"("function (open:0)"=T16."open or create", "file path"=w293) -> ("error out"=w285:errorcluster, "file size (bytes)"=w287:i32, "refnum"=w286:refnum<file>)  [unwired: 6 in, 1 out]
                n148 = Concatenate Strings(w306, w170, w298, w170, w307, w170, w308, w170, w275, w170, w274, w170, w309, w170, w310, w170, w299, w170, w313, w170, w311, w170, w312, w170, w300, w170, w301, w170, w302, w170, w303, w170, w304, w170, w272, w170, w263, w170, w195, w170, w262, w170, w261, w170, w252, w170, w251, w170, w250, w170, w249, w170, w246, w170, w245, w170, w234, w170, w233, w170, w232, w170, w231, w170, w224, w170, w223, w170, w222, w170, w221, w170, w214, w170, w213, w170, w212, w170, w211, w170, w210, w170, w209, w170, w208, w170, w207, w170, w206, w170, w205, w170, w204, w170, w203, w170, w202, w170, w201, w170, w200, w170, w199, w170, w182, w170, w181, w170, w198, w170, w194, w170, w193, w170, w192, w170, w191, w170, w190, w170, w189, w170, w188, w170, w187, w170, w186, w170, w185, w170, w184, w170, w183, w170, w180, w170, w179, w170, w178, w170, w177, w170, w169, w170, w168, "\n" ("string")) -> (w295:string)
                n149 = Set File Position(offset (in bytes) (0)=w287, refnum=w286, error in=w285) -> (refnum out=w290:refnum<file>, error out=w291:errorcluster)  [unwired: 1 in]
                n150 = Write to Binary File(file (use dialog)=w290, data=w295, error in=w291, 5:FALSE ("prepend array or string size? (T)")) -> (refnum out=w289:refnum<file>, error out=w288:errorcluster)  [unwired: 2 in, 1 out]
                n151 = Close File(refnum=w289, error in=w288) -> ()  [unwired: 2 out]
              }
              frame True {
                w315 = "\t" ("string")
                n152 = String To Path(string="C:\\frc\\templog.txt") -> (path=w379:path)
                n153 = call <vilib>:"Open_Create_Replace File.vi"("function (open:0)"=T16."open or create", "file path"=w379) -> ("error out"=w387:errorcluster, "file size (bytes)"=w385:i32, "refnum"=w386:refnum<file>)  [unwired: 6 in, 1 out]
                n154 = Set File Position(offset (in bytes) (0)=w385, refnum=w386, error in=w387) -> (refnum out=w382:refnum<file>, error out=w381:errorcluster)  [unwired: 1 in]
                n155 = Concatenate Strings("time" ("string"), w315, "Distance" ("string"), w315, "Camera X" ("string"), w315, "Camera Y" ("string"), w315, "Arm Encoder" ("string"), w315, "Shooter RPM", w315, "Left Front Drive Current" ("string"), w315, "Left Rear Drive Current" ("string"), w315, "Right Front Drive Current" ("string"), w315, "Right Rear Drive Current" ("string"), w315, "Pivot Left Current" ("string"), w315, "Pivot Right Current" ("string"), w315, "Roller Current" ("string"), w315, "Lift Left Current" ("string"), w315, "Lift Right Current" ("string"), w315, "Shoot Current" ("string"), w315, "Gear Shift Current", w315, "Total Current" ("string"), w315, "Total Power", w315, "PDP Temperature ", w315, "Screw Encoder SetPoint", w315, "Below Carry", w315, "Arm Encoder Speed", w315, "Screw Encoder Position", w315, "Arm Right Encoder Position", w315, "Screw Right Position", w315, "Arm PID SetPoint", w315, "Arm PID At SetPoint", w315, "Screw PID At SetPoint", w315, "Shooter Period", w315, "Shooter Status", w315, "Drive Encoder Distance", w315, "Drive Left Encoder Distance", w315, "Drive Right Encoder Distatnce", w315, "Drive Average Speed", w315, "Drive Left Speed", w315, "Drive Right Speed", w315, "Camera X", w315, "Driver A", w315, "Driver B", w315, "Driver X", w315, "Driver Y", w315, "Driver LB", w315, "Driver RB", w315, "Driver LT", w315, "Driver RT", w315, "Driver Start", w315, "Driver Back", w315, "Operator A", w315, "Operator B", w315, "Operator X", w315, "Operator Y", w315, "Operator LB", w315, "Operator RB", w315, "Operator LT", w315, "Operator RT", w315, "Operator Start", w315, "Operator Back", w315, "Auton Case", w315, "Auton Finished", "\n" ("string")) -> (w361:string)
                n156 = Write to Binary File(file (use dialog)=w382, data=w361, error in=w381, 5:FALSE ("prepend array or string size? (T)")) -> (refnum out=w383:refnum<file>, error out=w384:errorcluster)  [unwired: 2 in, 1 out]
                n157 = Close File(refnum=w383, error in=w384) -> ()  [unwired: 2 out]
              }
            }
          }
        }
        n158 = call "Prepare Joystick Data for Displays.vi"("Joystick Values"=w136) -> ("Buttons"=→"JS1 Buttons":T24, "Z Axis"=→"JS1 Z":dbl, "Cartesian Data"=→"JS1 Graph":cluster{"X axis":dbl, "X axis":dbl}[])  [unwired: 8 in]
        n159 = call "Prepare Joystick Data for Displays.vi"("Joystick Values"=w131) -> ("Buttons"=→"JS2 Buttons":T24, "Z Axis"=→"JS2 Z":dbl, "Cartesian Data"=→"JS2 Graph":cluster{"X axis":dbl, "X axis":dbl}[])  [unwired: 8 in]
        n160 = call-poly <vilib>:"NT Read Value.vi"("Name"="RobotDrive Motors") -> ("Numeric Array"=w126:dbl[])  [unwired: 9 in, 1 out]
        n161 = Index Array(array=w126, index #1=1, index #4=0) -> ()  [unwired: 2 in, 4 out]
        n162 = call-poly <vilib>:"NT Read Value.vi"("Name"="Auton Finished") -> ("Boolean"=→"Auton Finished 2":bool)  [unwired: 9 in, 1 out]
        n163 = call-poly <vilib>:"NT Read Value.vi"("Name"="Auton Finished") -> ("Boolean"=→"Auton Finished":bool)  [unwired: 9 in, 1 out]
      }
    }
  }
  n164 = while {
    tunnel: u16 1741 ("timeout ms (25000)") -> [w389]
    stop <- FALSE stop-if-true
    n165 = TCP Create Listener(10:w389) -> (0:w388:errorcluster, 3:w390:refnum<k5>)  [unwired: 4 in, 1 out]
    n166 = case shown="No Error" w388 {
      selector: w388 -> [w392 _]
      tunnel: w390 -> [w393 _]
      frame No Error {
        n167 = while {
          tunnel: w393 -> [w396]
          tunnel: w392 -> [w395]
          stop <- FALSE stop-if-true
          n168 = TCP Wait On Listener(8:w395, 11:w396) -> (0:w397:errorcluster, 4:w398:refnum<k5>)  [unwired: 2 in, 3 out]
          n169 = local write "TCP"(w398) -> ()
          n170 = case shown="No Error" w397 {
            frame No Error {
            }
            frame Error {
              n171 = Wait (ms)(milliseconds to wait=u32 1000) -> ()  [unwired: 1 out]
            }
          }
        }
      }
      frame Error {
        n172 = Wait (ms)(milliseconds to wait=u32 1000) -> ()  [unwired: 1 out]
      }
    }
  }
  n173 = while {
    tunnel: w60 -> [w418]
    tunnel: w59 -> [_]
    tunnel: [w419] -> _
    i -> [w419]
    stop <- FALSE stop-if-true
    # "Optionally read the DB image,\nlog, or retrieve images from a\nlogged match"
    n174 = case shown="True" "Camera Switch" {
      tunnel: ["Vision" w422] -> w409
      frame False {
      }
      frame True {
        n175 = call-poly <vilib>:"NT Read Value.vi"("Default Value"=FALSE, "Name"="Below Carry") -> ("Boolean"=w425:bool)  [unwired: 8 in, 1 out]
        n176 = case shown="True" w425 {
          tunnel: [u16 3 ("Vision") u16 2 ("Vision")] -> w422
          frame False {
          }
          frame True {
          }
        }
      }
    }
    n177 = call-poly <vilib>:"NT Read Value.vi"("Name"="Drive Angle at Setpoint") -> ("Boolean"=→"Shoot Now":bool)  [unwired: 9 in, 1 out]
    n178 = call-poly <vilib>:"NT Write Value.vi"("Numeric"="Defense Type", "Name"="Defense Type") -> ()  [unwired: 9 in, 1 out]
    n179 = local read "Camera IP"() -> (w412:string)
    n180 = local read "Rec Mode"() -> (w413:enum32{"Stop", "Record", "Playback"})
    n181 = call <vilib>:"WPI_CameraRead MJPG for Dashboard.vi"("Camera Settings"="Camera Settings", "Rec Mode"=w413, "Camera IP"=w412, "Camera Mode"=w409, "Refnum in"=w418) -> ("Active"=w416:bool, "Refnum out"=w417:T10, "FPS"=w415:dbl, "Bandwidth (Mbps)"=w411:dbl)  [unwired: 3 in]
    "Mbps" <- w411
    n182 = call-poly <vilib>:"NT Write Value.vi"("Boolean"="Shoot", "Name"="Shoot") -> ()  [unwired: 9 in, 1 out]
    n183 = case shown="True" w416 {
      tunnel: w417 -> [_ w522]
      tunnel: w411 -> [_ w521]
      tunnel: w415 -> [_ w520]
      frame False {
        w428 = u32 1985280 ("Color Box")
        # "Sleep for 500ms"
        n184 = Bundle("Color Box"=w428, "Color Box"=w428) -> (w430:cluster{"Color Box":u32, "Color Box":u32})  [unwired: 1 out]
        n185 = Build Array(w430) -> (w429:cluster{"Color Box":u32, "Color Box":u32}[])
        n186 = property on="Mbps LED" class="Bool (strict)"("Colors [4]"=w429) -> ()  [unwired: 2 in, 2 out]
        n187 = Wait Until Next ms Multiple(millisecond multiple=u32 500) -> ()  [unwired: 1 out]
      }
      frame True {
        # "Here is where you would annotate,\npossibly process, and display the image"
        # "Update Mbps LED"
        n188 = case shown="Default" w521 {
          tunnel: [u32 6618880 ("Color Box") u32 16776722 ("Color Box") u32 16716800 ("Color Box")] -> w523
          frame Default {
          }
          frame 4, 5 {
          }
          frame 6.. {
          }
        }
        n189 = call "IMAQ Clear Overlay"("Image"=w522) -> ("error out"=w526:errorcluster, "Image Out"=w519:T10)  [unwired: 2 in, 7 out]
        n190 = Unbundle By Name(w526) -> ("status"=w527:bool)
        n191 = call "FRC Color Processing Example.vi"("Std Devs for Calibration"="Std Devs for Calibration", "LED Color"="LED Color", "Min Score Threshold"="Min Score Threshold", "New Image"=w519, "Camera Type"="Camera Type") -> ("Detected Targets"=w476:T7, "Original Image"=→"Camera Image":T10)  [unwired: 5 in]
        "Detected Targets" <- w476
        n192 = property on="Image Message" class="Str"("Visible"=w527) -> ()  [unwired: 2 in, 2 out]
        n193 = Bundle("Color Box"=w523, "Color Box"=w523) -> (w525:cluster{"Color Box":u32, "Color Box":u32})  [unwired: 1 out]
        n194 = Array To Cluster(array=w476) -> (cluster=w514:T25)
        n195 = Build Array(w525) -> (w524:cluster{"Color Box":u32, "Color Box":u32}[])
        n196 = property on="Mbps LED" class="Bool (strict)"("Colors [4]"=w524) -> ()  [unwired: 2 in, 2 out]
        n197 = Unbundle(w514) -> ("Detected Targets[0]"=w513:T26, "Detected Targets[1]"=w489:T26, "Detected Targets[2]"=w477:T26)  [unwired: 6 out]
        n198 = Unbundle(w513) -> ("Distance (ft)"=w450:dbl, "Center"=w512:cluster{dbl, dbl}, "Normalized Rect"=w511:T27)
        n199 = Unbundle(w489) -> ("Distance (ft)"=w445:dbl, "Center"=w490:cluster{dbl, dbl}, "Normalized Rect"=w491:T27)
        n200 = Unbundle(w477) -> ("Distance (ft)"=w439:dbl, "Center"=w488:cluster{dbl, dbl}, "Normalized Rect"=w487:T27)
        n201 = Not Equal To 0?(x=w450) -> (x != 0?=w453:bool)
        n202 = Not Equal To 0?(x=w445) -> (x != 0?=w448:bool)
        n203 = Not Equal To 0?(x=w439) -> (x != 0?=w442:bool)
        n204 = Unbundle(w512) -> (w471:dbl)  [unwired: 1 out]
        n205 = Unbundle(w511) -> ("Numeric"=w503:dbl, "Numeric 2"=w470:dbl, "Numeric 3"=w501:dbl, "Numeric 5"=w505:dbl)
        n206 = Unbundle(w490) -> (w475:dbl)  [unwired: 1 out]
        n207 = Unbundle(w491) -> ("Numeric"=w498:dbl, "Numeric 2"=w469:dbl, "Numeric 3"=w500:dbl, "Numeric 5"=w496:dbl)
        n208 = Unbundle(w488) -> (w474:dbl)  [unwired: 1 out]
        n209 = Unbundle(w487) -> ("Numeric"=w480:dbl, "Numeric 2"=w468:dbl, "Numeric 3"=w478:dbl, "Numeric 5"=w482:dbl)
        n210 = Build Array(w471, w475, w474) -> (w472:dbl[])
        n211 = Build Array(w470, w469, w468) -> (w467:dbl[])
        n212 = Select(t=w450, s=w453, f=100.0) -> (s? t:f=w449:dbl)
        n213 = Select(t=w445, s=w448, f=100.0) -> (s? t:f=w444:dbl)
        n214 = Select(t=w439, s=w442, f=100.0) -> (s? t:f=w440:dbl)
        n215 = call-poly <vilib>:"NT Write Value.vi"("Numeric"=w475, "Name"="ImageXCenter1") -> ()  [unwired: 9 in, 1 out]
        n216 = call-poly <vilib>:"NT Write Value.vi"("Numeric"=w471, "Name"="ImageXCenter0") -> ()  [unwired: 9 in, 1 out]
        n217 = call-poly <vilib>:"NT Write Value.vi"("Numeric"=w505, "Name"="ImageBottom0") -> ()  [unwired: 9 in, 1 out]
        n218 = call-poly <vilib>:"NT Write Value.vi"("Numeric"=w496, "Name"="ImageBottom1") -> ()  [unwired: 9 in, 1 out]
        n219 = call-poly <vilib>:"NT Write Value.vi"("Numeric"=w474, "Name"="ImageXCenter2") -> ()  [unwired: 9 in, 1 out]
        n220 = call-poly <vilib>:"NT Write Value.vi"("Numeric"=w498, "Name"="ImageLeft1") -> ()  [unwired: 9 in, 1 out]
        n221 = call-poly <vilib>:"NT Write Value.vi"("Numeric"=w469, "Name"="ImageTop1") -> ()  [unwired: 9 in, 1 out]
        n222 = call-poly <vilib>:"NT Write Value.vi"("Numeric"=w503, "Name"="ImageLeft0") -> ()  [unwired: 9 in, 1 out]
        n223 = call-poly <vilib>:"NT Write Value.vi"("Numeric"=w470, "Name"="ImageTop0") -> ()  [unwired: 9 in, 1 out]
        n224 = call-poly <vilib>:"NT Write Value.vi"("Numeric"=w501, "Name"="ImageRight0") -> ()  [unwired: 9 in, 1 out]
        n225 = call-poly <vilib>:"NT Write Value.vi"("Numeric"=w500, "Name"="ImageRight1") -> ()  [unwired: 9 in, 1 out]
        n226 = call-poly <vilib>:"NT Write Value.vi"("Numeric"=w480, "Name"="ImageLeft2") -> ()  [unwired: 9 in, 1 out]
        n227 = call-poly <vilib>:"NT Write Value.vi"("Numeric"=w468, "Name"="ImageTop2") -> ()  [unwired: 9 in, 1 out]
        n228 = call-poly <vilib>:"NT Write Value.vi"("Numeric"=w478, "Name"="ImageRight2") -> ()  [unwired: 9 in, 1 out]
        n229 = call-poly <vilib>:"NT Write Value.vi"("Numeric"=w482, "Name"="ImageBottom2") -> ()  [unwired: 9 in, 1 out]
        n230 = Multiply(x=1.142, y=w449) -> (x*y=w455:dbl)
        n231 = Multiply(x=1.142, y=w444) -> (x*y=w461:dbl)
        n232 = Multiply(x=1.142, y=w440) -> (x*y=w458:dbl)
        n233 = Subtract(x=w455, y=1.0255) -> (x-y=w451:dbl)
        n234 = Subtract(x=w461, y=1.0255) -> (x-y=w446:dbl)
        n235 = Subtract(x=w458, y=1.0255) -> (x-y=w443:dbl)
        n236 = Build Array(w451, w446, w443) -> (w473:dbl[])
        n237 = call-poly <vilib>:"NT Write Value.vi"("Numeric"=w451, "Name"="distanceToTarget0") -> ()  [unwired: 9 in, 1 out]
        n238 = call-poly <vilib>:"NT Write Value.vi"("Numeric"=w446, "Name"="distanceToTarget1") -> ()  [unwired: 9 in, 1 out]
        n239 = call-poly <vilib>:"NT Write Value.vi"("Numeric"=w443, "Name"="distanceToTarget2") -> ()  [unwired: 9 in, 1 out]
        n240 = Array Max & Min(array=w473) -> (min value=w434:dbl, min index (indices)=w466:i32)  [unwired: 2 out]
        "Target Distance" <- w434
        n241 = Index Array(array=w472, index=w466) -> (element=w465:dbl)
        "Target X" <- w465
        n242 = Index Array(array=w467, index=w466) -> (element=→"Target Y":dbl)
        n243 = Less?(x=w434, y=15.0) -> (x < y?=w435:bool)
        n244 = In Range and Coerce(upper limit=-0.1525, x=w465, lower limit=-0.1725) -> (In Range?=w436:bool)  [unwired: 1 out]
        n245 = And(x=w436, y=w435) -> (x .and. y?=w433:bool)
        "Camera Aimed" <- w433
        n246 = call-poly <vilib>:"NT Write Value.vi"("Boolean"=w433, "Name"="CameraAimed") -> ()  [unwired: 9 in, 1 out]
        "fps" <- w520
      }
    }
    n247 = call-poly <vilib>:"NT Write Value.vi"("Numeric"="Defense Location", "Name"="Defense Location") -> ()  [unwired: 9 in, 1 out]
  }
  n248 = while {
    tunnel: w54 -> [w542]
    shift-right: [w541] -> _
    shift-left: w52 -> [w540]
    tunnel: [w539] -> _
    tunnel: w51 -> [w538]
    tunnel: w47 -> [w537]
    tunnel: w46 -> [w536]
    tunnel: w45 -> [_]
    tunnel: w41 -> [w535]
    tunnel: w6 -> [w534]
    tunnel: w4 -> [w533]
    shift-right: [w532] -> _
    shift-left: _ -> [w531]
    i -> [w539]
    stop <- FALSE stop-if-true
    n249 = event shown="[0] Timeout" {
      selector: w536 -> [_ _ _ _ _ _ _ _ _ _ _ _ _ _ _ _ _ _ _ _ _ _]
      dyn-events: [_ _ _ _ _ _ _ _ _ _ _ _ _ _ _ _ w843 _ _ _ _ _] -> _
      timeout: u32 60 ("milliseconds to wait") -> [_ _ _ _ _ _ _ _ _ _ _ _ _ _ _ _ _ _ _ _ _ _]
      tunnel: w538 -> [w555 _ _ _ _ _ _ _ _ _ _ _ _ _ _ _ _ _ _ _ _ _]
      tunnel: "Test Tree" -> [_ _ _ _ _ _ _ _ _ _ _ w806 w815 w818 w823 w832 _ _ _ _ _ _]
      tunnel: w542 -> [_ w593 _ _ _ _ _ _ _ w768 w799 _ _ _ _ _ _ _ _ _ _ _]
      tunnel: [w552 w592 w696 w702 w714 w726 w734 w740 w753 w767 w792 w805 w813 w817 w822 w831 w845 w861 w863 w871 w882 w887] -> w541
      tunnel: w540 -> [w552 w592 w696 w702 w714 w726 w734 w740 w753 w766 w792 w805 w813 w817 w822 w831 w845 w861 w863 w871 w882 w887]
      tunnel: w537 -> [_ _ _ _ _ _ _ _ _ _ _ _ _ _ _ _ w846 _ w866 _ _ _]
      tunnel: w535 -> [_ _ _ _ _ _ _ _ _ _ _ _ _ _ _ _ w841 _ _ _ _ _]
      tunnel: w534 -> [_ _ _ _ _ _ _ _ _ _ _ _ _ _ _ _ w837 _ _ _ _ _]
      tunnel: w533 -> [w547 _ _ _ w712 _ _ _ _ _ _ _ _ _ _ _ _ _ _ _ _ _]
      tunnel: [w546 w591 w695 w701 w710 w720 w731 w739 w752 w765 w791 w804 w812 w816 w821 w830 w836 w859 w862 w867 w875 w888] -> w532
      tunnel: w531 -> [w546 w591 w695 w701 w710 _ _ w739 w752 w765 w791 w804 w812 w816 w821 w830 w836 w859 w862 w867 w875 w888]
      event Timeout {
        n250 = event-data() -> ()  [unwired: 1 in, 1 out]
        n251 = local read "Mode"() -> (w549:T5)
        n252 = call <vilib>:"Connextion Info.vi"() -> ("Connected"=→"NT Connection":bool)  [unwired: 10 in, 1 out]
        n253 = case shown="\"Test\"" "Dashboard Tab" {
          tunnel: w555 -> [_ w569 _ _]
          tunnel: "/TestMode/Automatic/" ("Name Pattern") -> [_ w568 _ _]
          tunnel: T28 [{"Operation"=enum."Clear", "Color Box"=14013909}, {"Operation"=enum."Clear", "Color Box"=14013909}, {"Operation"=enum."Clear", "Color Box"=14013909}, {"Operation"=enum."Clear", "Color Box"=14013909}, {"Operation"=enum."Update", "Color Box"=14013909}, {"Operation"=enum."Update", "Color Box"=16777215}, {"Operation"=enum."Clear", "Color Box"=14013909}, {"Operation"=enum."Clear", "Color Box"=14013909}, {"Operation"=enum."Clear", "Color Box"=14013909}] -> [_ w561 _ w578]
          tunnel: w549 -> [_ w560 _ w577]
          tunnel: u32[] [15790320, 15790320, 15790320, 15790320, 16777215, 16777215, 15790320, 15790320, 15790320] -> [_ _ _ w583]
          tunnel: w547 -> [_ _ _ w571]
          frame "Custom", Default {
          }
          frame "Test" {
            w567 = -2 ("Active Item:Row Number")
            n254 = Index Array(array=w561, index=w560) -> (element=w562:T32)
            n255 = Unbundle(w562) -> ("Operation"=w563:enum16{"Update", "Clear"}, "Color Box"=w564:u32)
            n256 = call <vilib>:"NT Read and Format Entries as Tree.vi"("Operation"=w563, "Name Pattern"=w568, "Tree Refnum"=w569) -> ()  [unwired: 7 in, 2 out]
            n257 = property on="Test Tree" class="Tree (strict)"("Active Item Row Number"=w567, "ActiveColNum"=w567, "CellBG"=w564, "Active Item Row Number"=-1 ("Active Item:Row Number"), "CellBG"=u32 5789784 ("Color Box")) -> ()  [unwired: 2 in, 2 out]
          }
          frame "Variables" {
            n258 = control-ref of="Tree"() -> (w570:refnum<vi>)
            n259 = call <vilib>:"NT Read and Format Entries as Tree.vi"("Tree Refnum"=w570) -> ()  [unwired: 9 in, 2 out]
          }
          frame "Commands" {
            w579 = u32 5789784 ("Color Box")
            w580 = T33 {"Row"=-1, "Column"=-2} ("Active Cell:Active Cell")
            w582 = T33 {"Row"=-2, "Column"=-2} ("Active Cell:Active Cell")
            n260 = Index Array(array=w578, index=w577) -> (element=w576:T32)
            n261 = Index Array(array=w583, index=w577) -> (element=w581:u32)
            n262 = property on="Command Selection" class="MCListbox (strict)"("ActiveCell"=w582, "CellBG"=w581, "ActiveCell"=w580, "CellBG"=w579) -> ()  [unwired: 2 in, 2 out]
            n263 = property on="Command Params" class="Tbl (strict)"("Active Cell"=w582, "Cell BG Color"=w581, "Active Cell"=w580, "Cell BG Color"=w579) -> ()  [unwired: 2 in, 2 out]
            n264 = Unbundle(w576) -> ("Operation"=w575:enum16{"Update", "Clear"})  [unwired: 1 out]
            n265 = call <vilib>:"WPI_DashboardUpdate RPC Info.vi"("Operation"=w575) -> ("update"=w573:bool, "commands"=w572:string[][])  [unwired: 9 in]
            n266 = local read "Command Selection"() -> (w574:i32)
            n267 = property on="Command Selection" class="MCListbox (strict)"("ItemNames"=w572) -> ()  [unwired: 2 in, 2 out]
            n268 = call <vilib>:"WPI_DashboardUpdate Command Params.vi"("Update"=w573, "NewVal"=w574, "Commands"=w572, "Param Tbl"=w571) -> ()  [unwired: 7 in, 1 out]
          }
        }
        n269 = call <vilib>:"NT Read String.vi"("Name"="/TestMode/TestName") -> ("String"=w558:string)  [unwired: 9 in, 1 out]
        n270 = case shown="\"\"" w558 {
          tunnel: "/TestMode/TestProgress" ("Name") -> [w585 _]
          tunnel: "/TestMode/TestProgressText" ("Name") -> [w584 _]
          frame Default {
            n271 = call <vilib>:"NT Read Number.vi"("Name"=w585) -> ("Numeric"=w586:dbl)  [unwired: 9 in, 1 out]
            n272 = call <vilib>:"NT Read String.vi"("Name"=w584) -> ("String"=w587:string)  [unwired: 9 in, 1 out]
            n273 = Bundle("Numeric"=w586, "String"=w587) -> (→"Progress":cluster{"Numeric":dbl, "String":string})  [unwired: 1 in]
          }
          frame "" {
            n274 = local write "Test Name"(u16 0) -> ()
            n275 = property on="Progress" class="Clust (strict)"("Visible"=FALSE) -> ()  [unwired: 2 in, 2 out]
          }
        }
      }
      event "Test Tree": Value Change {
        # "Show appropriate\ncontrols"
        n276 = event-data() -> ("CtlRef"=w596:refnum<vi>, "NewVal"=w594:string)  [unwired: 1 in]
        n277 = call <vilib>:"WPI_UtilitiesGetTreeIOName.vi"("NewVal"=w594, "TreeControl in"=w596) -> ("I/O Name"=w597:string)  [unwired: 9 in]
        n278 = case shown="\"Analog Out\", \"Motor\", \"PWM\"" w597 {
          selector: w597 -> [_ w604 _ w626 w635 _]
          tunnel: w594 -> [_ _ w623 w625 _ w642]
          tunnel: w593 -> [_ _ _ _ _ w641]
          frame Default {
            w599 = FALSE ("Visible")
            w598 = FALSE ("Visible")
            n279 = property on="Test Slider" class="Slide (strict)"("Visible"=w599) -> ()  [unwired: 2 in, 2 out]
            n280 = property on="On/Off" class="Bool (strict)"("Visible"=w599) -> ()  [unwired: 2 in, 2 out]
            n281 = property on="Rev/Fwd" class="Clust (strict)"("Visible"=w599) -> ()  [unwired: 2 in, 2 out]
            n282 = property on="Test Ring" class="Ring (strict)"("Visible"=w598) -> ()  [unwired: 2 in, 2 out]
            n283 = property on="Motor" class="Clust (strict)"("Visible"=w598) -> ()  [unwired: 2 in, 2 out]
          }
          frame "Analog Out", "Motor", "PWM" {
            w605 = FALSE ("Visible")
            n284 = case shown="\"Analog Out\"" w604 {
              tunnel: [1.0 ("Value") -1.0 ("Value") 0.0 ("Value")] -> w603
              tunnel: [255.0 ("Value") 1.0 ("Value") 5.0 ("Value")] -> w602
              tunnel: [128.0 ("Value") 0.0 ("Value") 0.0 ("Value")] -> w601
              tunnel: [64.0 ("Value") 0.5 ("Value") 1.0 ("Value")] -> w600
              frame "PWM" {
              }
              frame "Motor", Default {
              }
              frame "Analog Out" {
              }
            }
            n285 = property on="Test Slider" class="Slide (strict)"("Visible"=w605) -> ()  [unwired: 2 in, 2 out]
            n286 = property on="Test Ring" class="Ring (strict)"("Visible"=w605) -> ()  [unwired: 2 in, 2 out]
            n287 = property on="On/Off" class="Bool (strict)"("Visible"=w605) -> ()  [unwired: 2 in, 2 out]
            n288 = property on="Rev/Fwd" class="Clust (strict)"("Visible"=w605) -> ()  [unwired: 2 in, 2 out]
            n289 = property on="Motor" class="Clust (strict)"("Visible"=TRUE) -> ()  [unwired: 2 in, 2 out]
            n290 = property on="Value" class="Slide (strict)"("Value"=w601, "Scale.Minimum"=w603, "Scale.Maximum"=w602, "Scale.Increment"=w600) -> ()  [unwired: 2 in, 2 out]
          }
          frame "Servo" {
            w621 = FALSE ("Visible")
            n291 = call <vilib>:"NT Read Number.vi"("Name"=w623) -> ("Numeric"=w622:dbl)  [unwired: 9 in, 1 out]
            n292 = property on="Motor" class="Clust (strict)"("Visible"=w621) -> ()  [unwired: 2 in, 2 out]
            n293 = property on="Test Ring" class="Ring (strict)"("Visible"=w621) -> ()  [unwired: 2 in, 2 out]
            n294 = property on="On/Off" class="Bool (strict)"("Visible"=w621) -> ()  [unwired: 2 in, 2 out]
            n295 = property on="Rev/Fwd" class="Clust (strict)"("Visible"=w621) -> ()  [unwired: 2 in, 2 out]
            n296 = property on="Test Slider" class="Slide (strict)"("Visible"=TRUE, "Scale.Maximum"=170.0 ("Scale.Range:Maximum")) -> ()  [unwired: 2 in, 2 out]
            n297 = local write "Test Slider"(w622) -> ()
          }
          frame "Relay", "Solenoid" {
            w624 = FALSE ("Visible")
            n298 = property on="Motor" class="Clust (strict)"("Visible"=w624) -> ()  [unwired: 2 in, 2 out]
            n299 = property on="Test Slider" class="Slide (strict)"("Visible"=w624) -> ()  [unwired: 2 in, 2 out]
            n300 = property on="Test Ring" class="Ring (strict)"("Visible"=w624) -> ()  [unwired: 2 in, 2 out]
            n301 = Search and Replace String(input string=w625, search string="/Value  **", replace string="/Direction") -> (result string=w631:string)  [unwired: 5 in, 3 out]
            n302 = call <vilib>:"NT Read String.vi"("Name"=w631) -> ("String"=w629:string)  [unwired: 9 in, 1 out]
            n303 = Equal?(x="Both directions", y=w629) -> (x = y?=w627:bool)
            n304 = property on="Rev/Fwd" class="Clust (strict)"("Visible"=w627) -> ()  [unwired: 2 in, 2 out]
            n305 = Not(x=w627) -> (.not. x?=w628:bool)
            n306 = property on="On/Off" class="Bool (strict)"("Visible"=w628, "Caption.Text"=w626) -> ()  [unwired: 2 in, 2 out]
          }
          frame "Compressor", "Digital Out" {
            w634 = FALSE ("Visible")
            # "Get direction and finish"
            n307 = property on="Test Ring" class="Ring (strict)"("Visible"=w634) -> ()  [unwired: 2 in, 2 out]
            n308 = property on="Motor" class="Clust (strict)"("Visible"=w634) -> ()  [unwired: 2 in, 2 out]
            n309 = property on="Test Slider" class="Slide (strict)"("Visible"=w634) -> ()  [unwired: 2 in, 2 out]
            n310 = property on="Rev/Fwd" class="Clust (strict)"("Visible"=FALSE) -> ()  [unwired: 2 in, 2 out]
            n311 = property on="On/Off" class="Bool (strict)"("Visible"=TRUE, "Caption.Text"=w635) -> ()  [unwired: 2 in, 2 out]
          }
          frame "Camera" {
            n312 = call <vilib>:"Get Last Path Segment.vi"("String in"=w642) -> ("String out"=w643:string)  [unwired: 10 in]
            n313 = property on="Rev/Fwd" class="Clust (strict)"("Visible"=FALSE) -> ()  [unwired: 2 in, 2 out]
            n314 = case shown="\"White Balance  **\"" w643 {
              tunnel: w642 -> [w649 w658 w667 w676 w685 _ w691]
              tunnel: w641 -> [w647 w655 w664 w673 w682 _ _]
              frame "Size  **" {
                n315 = Index Array(array=w647) -> (element=w646:cluster{string[]})  [unwired: 1 in]
                n316 = call <vilib>:"NT Read String.vi"("Name"=w649) -> ("String"=w648:string)  [unwired: 9 in, 1 out]
                n317 = property on="Test Slider" class="Slide (strict)"("Visible"=FALSE) -> ()  [unwired: 2 in, 2 out]
                n318 = property on="Test Ring" class="Ring (strict)"("Visible"=TRUE) -> ()  [unwired: 2 in, 2 out]
                n319 = Unbundle(w646) -> (w644:string[])
                n320 = Match First String(2:w644, 3:w648) -> (0:w645:i32)  [unwired: 1 out]
                n321 = property on="Test Ring" class="Ring (strict)"("Value"=w645, "Strings []"=w644) -> ()  [unwired: 2 in, 2 out]
              }
              frame "White Balance  **" {
                n322 = call <vilib>:"NT Read String.vi"("Name"=w658) -> ("String"=w657:string)  [unwired: 9 in, 1 out]
                n323 = Index Array(array=w655, index=1) -> (element=w656:cluster{string[]})
                n324 = property on="Test Slider" class="Slide (strict)"("Visible"=FALSE) -> ()  [unwired: 2 in, 2 out]
                n325 = property on="Test Ring" class="Ring (strict)"("Visible"=TRUE) -> ()  [unwired: 2 in, 2 out]
                n326 = Unbundle(w656) -> (w653:string[])
                n327 = Match First String(2:w653, 3:w657) -> (0:w652:i32)  [unwired: 1 out]
                n328 = property on="Test Ring" class="Ring (strict)"("Value"=w652, "Strings []"=w653) -> ()  [unwired: 2 in, 2 out]
              }
              frame "Exposure  **" {
                n329 = call <vilib>:"NT Read String.vi"("Name"=w667) -> ("String"=w666:string)  [unwired: 9 in, 1 out]
                n330 = Index Array(array=w664, index=2) -> (element=w665:cluster{string[]})
                n331 = property on="Test Slider" class="Slide (strict)"("Visible"=FALSE) -> ()  [unwired: 2 in, 2 out]
                n332 = property on="Test Ring" class="Ring (strict)"("Visible"=TRUE) -> ()  [unwired: 2 in, 2 out]
                n333 = Unbundle(w665) -> (w661:string[])
                n334 = Match First String(2:w661, 3:w666) -> (0:w662:i32)  [unwired: 1 out]
                n335 = property on="Test Ring" class="Ring (strict)"("Value"=w662, "Strings []"=w661) -> ()  [unwired: 2 in, 2 out]
              }
              frame "Exposure Priority  **" {
                n336 = call <vilib>:"NT Read String.vi"("Name"=w676) -> ("String"=w675:string)  [unwired: 9 in, 1 out]
                n337 = Index Array(array=w673, index=3) -> (element=w674:cluster{string[]})
                n338 = property on="Test Slider" class="Slide (strict)"("Visible"=FALSE) -> ()  [unwired: 2 in, 2 out]
                n339 = property on="Test Ring" class="Ring (strict)"("Visible"=TRUE) -> ()  [unwired: 2 in, 2 out]
                n340 = Unbundle(w674) -> (w670:string[])
                n341 = Match First String(2:w670, 3:w675) -> (0:w671:i32)  [unwired: 1 out]
                n342 = property on="Test Ring" class="Ring (strict)"("Value"=w671, "Strings []"=w670) -> ()  [unwired: 2 in, 2 out]
              }
              frame "Color Enable  **" {
                n343 = call <vilib>:"NT Read String.vi"("Name"=w685) -> ("String"=w684:string)  [unwired: 9 in, 1 out]
                n344 = Index Array(array=w682, index=4) -> (element=w683:cluster{string[]})
                n345 = property on="Test Slider" class="Slide (strict)"("Visible"=FALSE) -> ()  [unwired: 2 in, 2 out]
                n346 = property on="Test Ring" class="Ring (strict)"("Visible"=TRUE) -> ()  [unwired: 2 in, 2 out]
                n347 = Unbundle(w683) -> (w679:string[])
                n348 = Match First String(2:w679, 3:w684) -> (0:w680:i32)  [unwired: 1 out]
                n349 = property on="Test Ring" class="Ring (strict)"("Value"=w680, "Strings []"=w679) -> ()  [unwired: 2 in, 2 out]
              }
              frame Default {
                n350 = property on="Test Slider" class="Slide (strict)"("Visible"=FALSE) -> ()  [unwired: 2 in, 2 out]
                n351 = property on="Test Ring" class="Ring (strict)"("Visible"=FALSE) -> ()  [unwired: 2 in, 2 out]
              }
              frame "Brightness  **", "Color Level  **", "Compression  **", "FPS  **", "Sharpness  **" {
                n352 = call <vilib>:"NT Read Number.vi"("Name"=w691) -> ("Numeric"=w690:dbl)  [unwired: 9 in, 1 out]
                n353 = property on="Test Ring" class="Ring (strict)"("Visible"=FALSE) -> ()  [unwired: 2 in, 2 out]
                n354 = property on="Test Slider" class="Slide (strict)"("Visible"=TRUE, "Scale.Maximum"=100.0 ("Scale.Range:Maximum")) -> ()  [unwired: 2 in, 2 out]
                n355 = local write "Test Slider"(w690) -> ()
              }
            }
            n356 = property on="Motor" class="Clust (strict)"("Visible"=FALSE) -> ()  [unwired: 2 in, 2 out]
            n357 = property on="On/Off" class="Bool (strict)"("Visible"=FALSE) -> ()  [unwired: 2 in, 2 out]
          }
        }
        n358 = property on="Progress" class="Clust (strict)"("Visible"=FALSE) -> ()  [unwired: 2 in, 2 out]
      }
      event "Test Name": Mouse Enter {
        # "Populate the ring with the list of tests"
        n359 = event-data() -> ()  [unwired: 1 in, 1 out]
        n360 = call <vilib>:"NT Read String Array.vi"("Name"="/TestMode/TestList") -> ("String Array"=w700:string[])  [unwired: 9 in, 1 out]
        n361 = Build Array (concatenate)("Select the test to run...", w700) -> (w699:string[])
        n362 = property on="Test Name" class="Ring (strict)"("Strings []"=w699) -> ()  [unwired: 2 in, 2 out]
      }
      event "Test Name": Value Change {
        w703 = FALSE ("Visible")
        # "Tell the robot the test name to run"
        n363 = event-data() -> ("NewVal"=w707:u16)  [unwired: 1 in]
        n364 = property on="Test Name" class="Ring (strict)"() -> ("Strings []"=w708:string[])  [unwired: 2 in, 2 out]
        n365 = Index Array(array=w708, index=w707) -> (element=w706:string)
        n366 = local write "Progress"(T9 {"Test Progress"=0, "Test Progress Text"=""} ("Progress")) -> ()
        n367 = property on="Progress" class="Clust (strict)"("Visible"=TRUE) -> ()  [unwired: 2 in, 2 out]
        n368 = property on="Test Ring" class="Ring (strict)"("Visible"=w703) -> ()  [unwired: 2 in, 2 out]
        n369 = property on="Motor" class="Clust (strict)"("Visible"=w703) -> ()  [unwired: 2 in, 2 out]
        n370 = property on="Test Slider" class="Slide (strict)"("Visible"=w703) -> ()  [unwired: 2 in, 2 out]
        n371 = property on="On/Off" class="Bool (strict)"("Visible"=w703) -> ()  [unwired: 2 in, 2 out]
        n372 = property on="Rev/Fwd" class="Clust (strict)"("Visible"=w703) -> ()  [unwired: 2 in, 2 out]
        n373 = call <vilib>:"NT Write String.vi"("String"=w706, "Name"="/TestMode/TestName") -> ()  [unwired: 9 in, 1 out]
      }
      event "Command Selection": Value Change {
        # "Get the params and show in table"
        n374 = event-data() -> ("NewVal"=w713:i32)  [unwired: 1 in]
        n375 = property on="Command Selection" class="MCListbox (strict)"() -> ("ItemNames"=w711:string[][])  [unwired: 2 in, 2 out]
        n376 = call <vilib>:"WPI_DashboardUpdate Command Params.vi"("NewVal"=w713, "Commands"=w711, "Param Tbl"=w712) -> ()  [unwired: 8 in, 1 out]
      }
      event "Execute Command": Value Change {
        # "Started one, Unique ID holds\nresponse"
        n377 = event-data() -> ()  [unwired: 1 in, 1 out]
        n378 = property on="Command Selection" class="MCListbox (strict)"() -> ("ItemNames"=w725:string[][])  [unwired: 2 in, 2 out]
        n379 = Index Array(array=w725, index (row)="Command Selection", index (col)=0) -> (element=w723:string)
        n380 = call <vilib>:"Invoke Commands.vi"("Command Params"="Command Params", "Function Name"=w723) -> ("Params"=w719:u8, "Started"=w718:bool)  [unwired: 7 in, 1 out]
        n381 = Array Subset(array="Command Params", length (row)=w719) -> (w720:string[][])  [unwired: 3 in]
        n382 = Select(t="Executing" ("Cmd Status"), s=w718, f="" ("Cmd Status")) -> (s? t:f=→"Cmd Status":string)
      }
      event "Command Selection": Double Click {
        n383 = event-data() -> ("Row"=w735:i32)  [unwired: 1 in]
        n384 = property on="Command Selection" class="MCListbox (strict)"() -> ("ItemNames"=w738:string[][])  [unwired: 2 in, 2 out]
        n385 = local read "Command Params"() -> (w733:string[][])
        n386 = Index Array(array=w738, index (row)=w735, index (col)=0) -> (element=w736:string)
        n387 = call <vilib>:"Invoke Commands.vi"("Command Params"=w733, "Function Name"=w736) -> ("Params"=w732:u8, "Started"=w727:bool)  [unwired: 7 in, 1 out]
        n388 = Array Subset(array=w733, length (row)=w732) -> (w731:string[][])  [unwired: 3 in]
        n389 = Select(t="Executing" ("Cmd Status"), s=w727, f="" ("Cmd Status")) -> (s? t:f=w728:string)
        n390 = local write "Cmd Status"(w728) -> ()
      }
      event "CheckList": Double Click {
        # "Shift clears all"
        # "Update symbols on the listbox"
        n391 = event-data() -> ("PlatMods.Shift"=w741:bool, "Row"=w743:i32)  [unwired: 1 in]
        n392 = case shown="True" w741 {
          tunnel: w743 -> [w747 _]
          tunnel: 1 -> [w746 _]
          frame False {
            n393 = property on="CheckList" class="LstBox (strict)"() -> ("Item Symbols"=w745:i32[])  [unwired: 2 in, 2 out]
            n394 = Replace Array Subset(array=w745, new element=w746, index=w747) -> (w744:i32[])
            n395 = property on="CheckList" class="LstBox (strict)"("Item Symbols"=w744) -> ()  [unwired: 2 in, 2 out]
          }
          frame True {
            w748 = 0 ("Top Row")
            n396 = property on="CheckList" class="LstBox (strict)"() -> ("Number of Rows"=w750:u32)  [unwired: 2 in, 2 out]
            n397 = Initialize Array(0, w750) -> (w749:i32[])
            n398 = property on="CheckList" class="LstBox (strict)"("Top Row"=w748, "Value"=w748, "Item Symbols"=w749) -> ()  [unwired: 2 in, 2 out]
          }
        }
      }
      event "CheckList": Key Down {
        # "Update symbols on the listbox\nLeft and right keys check and uncheck"
        n399 = event-data() -> ("VKey"=w755:T29)  [unwired: 1 in]
        n400 = case shown="\"Left\", \"Right\"" w755 {
          selector: w755 -> [w760 _]
          tunnel: eventvkey."Left" ("VKey") -> [w758 _]
          frame "Left", "Right" {
            n401 = Equal?(x=w758, y=w760) -> (x = y?=w759:bool)
            n402 = Select(t=0, s=w759, f=1) -> (s? t:f=w761:i32)
            n403 = property on="CheckList" class="LstBox (strict)"() -> ("Item Symbols"=w764:i32[])  [unwired: 2 in, 2 out]
            n404 = Replace Array Subset(array=w764, new element=w761, index="CheckList") -> (w763:i32[])
            n405 = property on="CheckList" class="LstBox (strict)"("Item Symbols"=w763) -> ()  [unwired: 2 in, 2 out]
          }
          frame Default {
          }
        }
      }
      event "DB Camera Config": Value Change {
        # "Show or hide the cluster of controls, store in ini file"
        n406 = event-data() -> ("NewVal"=w769:bool)  [unwired: 1 in]
        n407 = case shown="False" w769 {
          tunnel: w768 -> [w778 _]
          tunnel: [w771 w789] -> w767
          tunnel: w766 -> [w770 w789]
          frame False {
            w785 = "Camera"
            w788 = FALSE ("Visible")
            n408 = Index Array(array=w778) -> (element=w781:cluster{string[]})  [unwired: 1 in]
            n409 = property on="Camera Settings" class="Clust (strict)"("Visible"=w788) -> ()  [unwired: 2 in, 2 out]
            n410 = local write "DB Camera Config"(w788) -> ()
            n411 = Unbundle(w781) -> (w780:string[])
            n412 = local read "Camera Settings"() -> (w777:T4)
            n413 = Unbundle(w777) -> ("Frame Rate"=w776:i32, "Compression"=w775:i32, "Size"=w779:u16)
            n414 = Index Array(array=w780, index=w779) -> (element=w774:string)
            n415 = call-poly <vilib>:"Write Key.vi"("section"=w785, "value"=w774, "key"="Size", "refnum"=w770) -> ("refnum out"=w787:T15)  [unwired: 2 in, 5 out]
            n416 = call-poly <vilib>:"Write Key.vi"("section"=w785, "value"=w776, "key"="FrameRate", "refnum"=w787) -> ("refnum out"=w786:T15)  [unwired: 1 in, 6 out]
            n417 = call-poly <vilib>:"Write Key.vi"("section"=w785, "value"=w775, "key"="Compression", "refnum"=w786) -> ("refnum out"=w772:T15)  [unwired: 1 in, 6 out]
            n418 = call <vilib>:"Close Config Data.vi"("refnum"=w772) -> ("file path"=w773:path)  [unwired: 2 in, 8 out]
            n419 = call <vilib>:"Open Config Data.vi"("configuration file path"=w773) -> ("refnum"=w771:T15)  [unwired: 8 in, 2 out]
          }
          frame True {
            n420 = property on="Camera Settings" class="Clust (strict)"("Visible"=TRUE) -> ()  [unwired: 2 in, 2 out]
          }
        }
      }
      event "Camera Settings": Value Change {
        # "Update summary string when any elements of DB camera change"
        n421 = event-data() -> ("NewVal"=w803:T4)  [unwired: 1 in]
        n422 = Index Array(array=w799) -> (element=w798:cluster{string[]})  [unwired: 1 in]
        n423 = Unbundle(w803) -> ("Frame Rate"=w794:i32, "Compression"=w793:i32, "Size"=w796:u16)
        n424 = Unbundle(w798) -> (w797:string[])
        n425 = Index Array(array=w797, index=w796) -> (element=w795:string)
        n426 = Format Into String(format string="%s   %dfps   %d%%", w795, w794, w793) -> (resulting string=w800:string)  [unwired: 2 in, 1 out]
        n427 = Build Array(w800) -> (w801:string[])
        n428 = property on="DB Camera Config" class="Bool (strict)"("Strings [4]"=w801) -> ()  [unwired: 2 in, 2 out]
      }
      event "Motor.Enable": Value Change {
        # "When the test mode otor enable helper is set, update that\ntree row item's value"
        n429 = event-data() -> ("NewVal"=w810:bool)  [unwired: 1 in]
        n430 = Unbundle("Motor") -> ("Value"=w809:dbl)  [unwired: 1 out]
        n431 = Select(t=w809, s=w810, f=0.0) -> (s? t:f=w807:dbl)
        n432 = call <vilib>:"NT Write Number.vi"("Numeric"=w807, "Name"=w806) -> ()  [unwired: 9 in, 1 out]
      }
      event "Test Slider": Value Change {
        # "When the test mode slider helper is set, update that\ntree row item's value"
        n433 = event-data() -> ("NewVal"=w814:dbl)  [unwired: 1 in]
        n434 = call <vilib>:"NT Write Number.vi"("Numeric"=w814, "Name"=w815) -> ()  [unwired: 9 in, 1 out]
      }
      event "On/Off": Value Change {
        # "When the test mode on/off helper value is set, update that\ntree row item's value"
        n435 = event-data() -> ("NewVal"=w820:bool)  [unwired: 1 in]
        n436 = Boolean To (0,1)(Boolean=w820) -> (0, 1=w819:i16)
        n437 = call <vilib>:"NT Write Number.vi"("Numeric"=w819, "Name"=w818) -> ()  [unwired: 9 in, 1 out]
      }
      event "Rev/Fwd": Value Change {
        # "When the test mode helper value for relays is set, update that\ntree row item's value"
        n438 = event-data() -> ("NewVal.Forward"=w829:bool, "NewVal.Reverse"=w828:bool)  [unwired: 1 in]
        n439 = Boolean To (0,1)(Boolean=w829) -> (0, 1=w825:i16)
        n440 = Boolean To (0,1)(Boolean=w828) -> (0, 1=w827:i16)
        n441 = Negate(x=w827) -> (-x=w826:i16)
        n442 = Add(x=w825, y=w826) -> (x+y=w824:i16)
        n443 = call <vilib>:"NT Write Number.vi"("Numeric"=w824, "Name"=w823) -> ()  [unwired: 9 in, 1 out]
      }
      event "Test Ring": Value Change {
        # "When a test mode helper value is selected from the ring,\nset the tree item's variable to the string value"
        n444 = event-data() -> ("NewVal"=w834:u16)  [unwired: 1 in]
        n445 = property on="Test Ring" class="Ring (strict)"() -> ("Strings []"=w835:string[])  [unwired: 2 in, 2 out]
        n446 = Index Array(array=w835, index=w834) -> (element=w833:string)
        n447 = call <vilib>:"NT Write String.vi"("String"=w833, "Name"=w832) -> ()  [unwired: 9 in, 1 out]
      }
      event "Rec Mode": Value Change {
        # "Update globals for recording mode and path to read log from.\nClear when logging and let NetworkTables set path for vision to\nuse."
        n448 = event-data() -> ("NewVal"=w847:enum32{"Stop", "Record", "Playback"})  [unwired: 1 in]
        n449 = global write "WPI_DashboardLogging Global.vi" "Recording"(w847) -> ()
        n450 = global write "WPI_DashboardLogging Global.vi" "Logging Filename"(path "") -> ()
        n451 = case shown="\"Playback\"" w847 {
          tunnel: w846 -> [_ w849 w858]
          tunnel: [_ _ w857] -> w843
          tunnel: [_ _ w856] -> _
          tunnel: w841 -> [_ _ w854]
          tunnel: cluster{i32, i32} {-250, 170} -> [_ _ w853]
          tunnel: [_ _ T30 {"Image Size"=TRUE, "Image Type"=TRUE, "Pixel Value"=TRUE, "ROI Information"=TRUE, "Zoom Factor"=FALSE} ("Image Information Shown:All Elements")] -> w839
          tunnel: [_ _ TRUE ("Zoom Factor")] -> w838
          tunnel: w837 -> [_ _ w850]
          frame Default {
          }
          frame "Stop", "Record" {
            # "Place Window too"
            n452 = invoke class="VI" method="FP.Close"(reference=w849) -> (reference out=w848:refnum<vi>)  [unwired: 2 in, 2 out]
            n453 = invoke class="VI" method="Abort VI"(reference=w848) -> ()  [unwired: 2 in, 3 out]
          }
          frame "Playback" {
            n454 = call "Open Playback Panel.vi"("Offset"=w853, "DB VI Ref"=w854, "Playback in"=w858) -> ("Playback out"=w855:refnum<vi>)  [unwired: 8 in]
            n455 = register-events(w855, w850) -> (reference out=w857:refnum<event-registration>, error out=w856:errorcluster)  [unwired: 2 in]
          }
        }
        n456 = call <vilib>:"WPI_DashboardNT Log FieldName Cache.vi"("Operation"=enum16{"Lookup/Add", "Index", "Clear"}."Clear") -> ()  [unwired: 8 in, 3 out]
        n457 = property on="Camera Image" class="ImageControl"("Image Information Shown"=w839, "Image Information Visible"=w838) -> ()  [unwired: 2 in, 2 out]
      }
      event Panel Close {
        w860 = enum32{"Stop", "Record", "Playback"}."Stop" ("Rec Mode")
        # "Playback window has been closed, abort"
        n458 = event-data() -> ()  [unwired: 1 in, 4 out]
        n459 = local write "Rec Mode"(w860) -> ()
        n460 = global write "WPI_DashboardLogging Global.vi" "Recording"(w860) -> ()
      }
      event Panel Close {
        # "Abort playback window and ourself"
        n461 = event-data() -> ()  [unwired: 1 in, 4 out]
        n462 = invoke class="VI" method="FP.Close"(reference=w866) -> (reference out=w865:refnum<vi>)  [unwired: 2 in, 2 out]
        n463 = invoke class="VI" method="Abort VI"(reference=w865) -> (error out=w864:errorcluster)  [unwired: 2 in, 2 out]
        n464 = invoke class="VI" method="Abort VI"(error in=w864) -> ()  [unwired: 2 in, 3 out]
      }
      event User Event {
        n465 = event-data() -> ("IDs"=w874:cluster{"RPC field ID":u16, "Unique ID":u16}, "String"=w873:string)  [unwired: 1 in]
        n466 = Bundle("IDs"=w874, "String"=w873) -> (w872:T11)  [unwired: 1 in]
        n467 = call <vilib>:"Retrieve RPC Response.vi"("RPC Response"=w872) -> ("Output"=w869:string[][])  [unwired: 10 in]
        n468 = Build Array (concatenate)(w867, w869) -> (w868:string[][])
        n469 = local write "Command Params"(w868) -> ()
        n470 = local write "Cmd Status"("" ("Cmd Status")) -> ()
      }
      event "Vision": Value Change {
        # "Enable/Disable Compression slider.\nHW USB is hard-coded into the camera"
        n471 = event-data() -> ("NewVal"=w881:u16)  [unwired: 1 in]
        n472 = Equal?(x=w881, y=u32 2 ("milliseconds to wait")) -> (x = y?=w879:bool)
        n473 = Select(t=T31."Disabled and Grayed Out" ("Disabled"), s=w879, f=T31."Enabled" ("Disabled")) -> (s? t:f=w876:T31)
        n474 = property on="Compression" class="Slide (strict)"("DisabledEnum"=w876) -> ()  [unwired: 2 in, 2 out]
      }
      event "Tree": Double Click {
        n475 = event-data() -> ("PlatMods"=w886:T34, "Tag"=w885:string)  [unwired: 1 in]
        n476 = Unbundle(w886) -> ("Shift"=w884:bool)  [unwired: 4 out]
        n477 = Not(x=w884) -> (.not. x?=w883:bool)
        n478 = call <vilib>:"NT Update Persistence.vi"("Persistence"=w883, "Name"=w885) -> ()  [unwired: 9 in, 1 out]
      }
    }
  }
  n479 = local write "Dashboard Tab"(T2."Drive" ("Dashboard Tab")) -> ()
  n480 = property on="On/Off" class="Bool (strict)"("Visible"=w16) -> ()  [unwired: 2 in, 2 out]
  n481 = property on="Motor" class="Clust (strict)"("Visible"=w16) -> ()  [unwired: 2 in, 2 out]
  n482 = property on="Progress" class="Clust (strict)"("Visible"=w16) -> ()  [unwired: 2 in, 2 out]
  n483 = property on="Test Ring" class="Ring (strict)"("Visible"=w16) -> ()  [unwired: 2 in, 2 out]
  n484 = property on="Rev/Fwd" class="Clust (strict)"("Visible"=w16) -> ()  [unwired: 2 in, 2 out]
  n485 = property on="Camera Settings" class="Clust (strict)"("Visible"=w16) -> ()  [unwired: 2 in, 2 out]
  n486 = local write "DB Camera Config"(w16) -> ()
  n487 = local write "Command Params"(string[][] [] ("Command Params")) -> ()
  n488 = global write "WPI_DashboardLogging Global.vi" "Recording"(w42) -> ()
  n489 = local write "Rec Mode"(w42) -> ()
  n490 = local write "Command Selection"(u16 0 ("milliseconds to wait")) -> ()
